vi "4ChNCS_BIOPAC_Zijing.vi"() -> ()   [LabVIEW 2016]
uses:
  <instrlib>/niUSRP/niUSRP Timestamp.ctl
  <vilib>/Utility/miscctls.llb/LVDateTimeRec.ctl
  <vilib>/Analysis/3filter.llb/Filter Passband Type.ctl
  <vilib>/sound2/lvsound2.llb/Sampling Mode.ctl
  <instrlib>/niUSRP/niUSRP Configure Time Start Trigger.vi
  <vilib>/Platform/browser.llb/Open URL in Default Browser (string).vi
  <instrlib>/niUSRP/niUSRP Write Tx Data (2D CDB).vi
  <instrlib>/niUSRP/niUSRP Fetch Rx Data (2D CDB).vi
  <vilib>/Analysis/3filter.llb/Butterworth Filter (DBL).vi
  <vilib>/Analysis/3filter.llb/Butterworth Filter (CDB).vi
  <vilib>/sound2/lvsound2.llb/Sound File Info (path).vi
  <vilib>/sound2/lvsound2.llb/Sound File Read Open.vi
  <vilib>/sound2/lvsound2.llb/Sound File Read (DBL).vi
  <vilib>/sound2/lvsound2.llb/Sound Output Write (DBL).vi
  <vilib>/measure/NI_MABase.lvlib
  <vilib>/Analysis/NI_AALBase.lvlib
  C:/Program Files (x86)/BIOPAC Systems, Inc/BIOPAC Hardware API 2.2 Education/x64/mpdev.dll
panel:
  in  "Mute":bool
  out "Play Sound":bool=TRUE
  in  "bottom filter":T1
  in  "top filter":T1=enum."Bandpass"
  out "Acq Started":bool
  out "# BIO View Q":i32
  out "# BIO Buffer":i32
  out "Boolean":bool=TRUE
  out "Disconnecting":bool
  out "Stopping":bool
  out "Connecting":bool
  out "Disconnected":bool
  in  "Show BIO":bool
  out "# BIOViewQ2":i32
  out "Array 1 View":dbl[](graph)
  out "Array 2 View":dbl[](graph)
  out "Array 3 View":dbl[](graph)
  out "Array 4 View":dbl[](graph)
  out "View Array Size":i32
  out "# Elements in Array":i32
  out "ACQ -# Elements":i32
  out "Receive Success":bool
  out "# ACQ cycles":i32
  out "Bytes Read":i32
  out "Bytes To Read":i32
  out "Receive Total Size":dbl format="%#_13g"
  out "Receiving":bool
  in  "Start Acquisition":bool
  in  "Disconnect":bool
  out "ACQ ms":dbl=250.0 format="%#_13g"
  in  "Stop Acquisition":bool
  out "Connected":bool
  in  "Sample Rate":dbl=1.0 caption="ms/sample" min=0.0
  in  "Analog Channels":i32[](array[numeric])=[1, 1, 1, 1]
  out "# Channels":dbl format="%#_13g"
  out "BIO Connect":i32
  in  "BIO Connect":bool=TRUE
  in  "OpenHTML":bool=TRUE
  in  "Abd (cm)":string="0"
  in  "Thorax (cm)":string="0"
  in  "Comments":string
  in  "Weight (lbs)":string="0"
  in  "Age (yrs)":string="0"
  in  "Sex":string(combo)="Female"
  in  "Height (cm)":string="0"
  in  "Case #":string="14"
  out "Start Time":T2
  out "Total Routine Time":dbl(slide) scale=0.0..300.0
  out "Elapsed Time":dbl caption="Elapsed Time (s)"
  out "Next Instruction":string
  out "Current Instruction":string
  in  "Routine Selection":T3(ring)
  out "Current Routine":string
  out "Tx3Rx4":dbl[](graph)
  out "Tx4Rx4":dbl[](graph)
  out "Tx4Rx3":dbl[](graph)
  out "Tx3Rx3":dbl[](graph)
  out "ChAmp":dbl[][](array[numeric])=[[1.7262327066457893e-05, 1.899698926539768e-05, 2.131979680782845e-05, 2.7507513862708948e-05, 3.236234947998919e-05, 3.384280863448985e-05, 3.3113712649913256e-05, 2.8744318806479064e-05, 2.4117959107532184e-05, 2.0714217164135817e-05, 1.7964639969242282e-05, 1.4127881869429752e-05, 1.5692535768228094e-05, 2.4152619914305532e-05, 2.8339686382715385e-05, 2.606906286720416e-05, 2.1755918570529384e-05, 2.0929028564145826e-05, 2.2419410493859248e-05, 2.1786896096171967e-05, 1.7145005999174206e-05, 1.5886785364638103e-05, 1.995380091360238e-05, 1.96084446445408e-05, 1.3881312052638574e-05, 5.368463432831762e-06, 7.886976522489036e-06, 1.718108126568357e-05, 1.984430714817916e-05, 1.8874058751572535e-05, 1.7869312672433515e-05, 1.7356735499504872e-05, 2.065235332503479e-05, 2.1951680154988656e-05, 2.0363547237431346e-05, 2.1229264430323524e-05, 2.188656276617781e-05, 2.1477411495382004e-05, 1.913194947952161e-05, 1.374906879007994e-05, 1.084407557924396e-05, 1.0538448835067238e-05, 1.3462486513328936e-05, 1.979383250422823e-05, 2.381539261154395e-05, 2.2167223174073578e-05, 1.7644503717147575e-05, 1.870536234643517e-05, 2.2751950524913166e-05, 2.340432192813861e-05, 2.2468849270761083e-05, 2.4188550691353842e-05, 2.7519058552290856e-05, 3.1102581077866726e-05, 3.580393911829494e-05, 3.78912649503874e-05, 3.327873597801261e-05, 2.4510981949940783e-05, 1.8465065354817837e-05, 1.7132224969133005e-05, 1.7642310138371268e-05, 1.88142956741822e-05, 1.560032046277488e-05, 9.753217862235494e-06, 1.2015090850038981e-05, 1.776834560720681e-05, 2.4803861691952522e-05, 2.8043624192078222e-05, 2.684382525540612e-05, 2.3530222840588965e-05, 2.0528849124310057e-05, 1.9668374613316667e-05, 1.9146637114645684e-05, 1.5474488036915515e-05, 1.739488550213199e-05, 2.5095299380068926e-05, 3.2858145215540916e-05, 3.439509649081835e-05, 2.6143868318774837e-05, 1.7977385637690134e-05, 1.6384181575586158e-05, 1.4888284293264162e-05, 1.1597491470576354e-05, 1.1445555578759772e-05, 1.4980688444081562e-05, 1.909173519498907e-05, 1.9461150455264684e-05, 1.845876729070065e-05, 1.8005010185132642e-05, 1.9028924898462435e-05, 1.7575955788217445e-05, 1.4184298105937452e-05, 9.414371560237339e-06, 5.4356042784590255e-06, 8.10928562517548e-06, 9.28876849225871e-06, 8.695785214389758e-06, 1.2695777397634576e-05, 1.6809431598631123e-05, 2.1908643727461497e-05], [0.39904903865563796, 0.39903176051530775, 0.39902405260596024, 0.3990221650023599, 0.3990182934858042, 0.39901299641778676, 0.39900459263010085, 0.39899398548309095, 0.3989851312683333, 0.3989817758172843, 0.39898441600096285, 0.3989920701551657, 0.3989957319087615, 0.3989970252526829, 0.3990014639144786, 0.3990082495650084, 0.39901677157837184, 0.39902202434845035, 0.3990170521098724, 0.3990061914814684, 0.39899957115083645, 0.39900163440594105, 0.39901134932465093, 0.3990245430143365, 0.3990299364956871, 0.3990206423396574, 0.39901294696264844, 0.399015237964853, 0.3990195320664335, 0.3990239908891069, 0.39902678858482366, 0.3990303142377581, 0.3990363654196349, 0.39903798034344395, 0.39903568308022536, 0.3990295778239386, 0.3990213145612541, 0.3990115641317417, 0.3990031911721688, 0.3990044335692754, 0.3990142055365442, 0.3990231880559529, 0.3990294810791408, 0.39903152543597487, 0.3990303417237137, 0.39902587131491124, 0.39902317862698444, 0.3990231908517323, 0.3990187535042287, 0.39901147460102687, 0.39900466569609977, 0.399000198693456, 0.398994572076958, 0.39898792975360287, 0.39898351183081265, 0.39898252129559103, 0.3989860199605185, 0.3989908704807006, 0.39899345184972185, 0.39899268675930705, 0.39898929894357515, 0.39898974479144206, 0.3989970434213525, 0.39900457970685, 0.3990084272376425, 0.3990059437407563, 0.39900092658003017, 0.3989998521554356, 0.3989999155043143, 0.39900335732390085, 0.3990086633280822, 0.39901161043288735, 0.3990153435576799, 0.3990232290578827, 0.39902895125044885, 0.3990233171970213, 0.39901091768095076, 0.3989963560226853, 0.3989823146041765, 0.39898013105698543, 0.39899131681473166, 0.3990088743561722, 0.39902163871137375, 0.39902552269435965, 0.3990216751013488, 0.3990108271690995, 0.3989999368161602, 0.39899179748001445, 0.3989869444795569, 0.3989823014007489, 0.3989811018380635, 0.3989866085692465, 0.3989974881575293, 0.399009653455826, 0.39902039237597164, 0.39903113834388676, 0.39903799466445666, 0.39903656085835637, 0.39902912933239515, 0.3990196685727854], [0.5089284260094796, 0.5089413529092005, 0.5089385924023097, 0.5089461735853302, 0.5089333321440155, 0.5089367652503622, 0.5089376331435306, 0.5089306671430541, 0.508949239645895, 0.5089486561361645, 0.5089529378833244, 0.5089419476875585, 0.5089298840108731, 0.5089475772042052, 0.5089441426339854, 0.5089427381450184, 0.5089483329108746, 0.5089280151098653, 0.5089336602793385, 0.5089062019851882, 0.5089074628030626, 0.5088932174425751, 0.5088701289561509, 0.5088760830698362, 0.5088683341509143, 0.5088818393635381, 0.5089000365985035, 0.5088962730652971, 0.5089053012825656, 0.5088919060061875, 0.5088858810710211, 0.5088778714303226, 0.508862396898039, 0.5088799706522465, 0.508890020250467, 0.5089068411749241, 0.508910151200762, 0.5088879724716624, 0.5088963605339264, 0.5088989546591678, 0.5089079531975655, 0.5089307483176185, 0.5089353690581762, 0.5089322510910641, 0.5089226818391756, 0.5089231205950179, 0.5089421889187917, 0.5089302121637822, 0.5089288553338916, 0.5089136387417116, 0.5088923938634197, 0.5088806790242092, 0.5088543127997475, 0.5088388632427274, 0.5088290815518671, 0.5088136498514574, 0.508828716232115, 0.5088373004254244, 0.5088536031198835, 0.5088663652543981, 0.5088663647379902, 0.5088663839922184, 0.5088589552438861, 0.5088642449634635, 0.5088725023266256, 0.5088718014416865, 0.5088674063260687, 0.5088515437004615, 0.5088682831786894, 0.5088713788197812, 0.5088809924897628, 0.508878513506942, 0.5088771181893693, 0.5088848435184512, 0.5088770842370816, 0.5088914766511436, 0.5089003523667647, 0.5089066301516674, 0.5089314320882471, 0.5089402101447223, 0.508962553406896, 0.5089753861787446, 0.5089593307295952, 0.5089478542324088, 0.5089278310589712, 0.5089248500720587, 0.5089163513653545, 0.5089005689237424, 0.5089083211616405, 0.5088993300683022, 0.5088927412237987, 0.5088830866377116, 0.5088718481995638, 0.5088897909905771, 0.5088809733102648, 0.5088790935282286, 0.5088680814653207, 0.5088523600270333, 0.5088613943195607, 0.5088543176402154], [2.0662941946213977e-05, 2.282608405319783e-05, 2.237600508813514e-05, 2.2542693256186783e-05, 2.041826329305299e-05, 1.6288400811782785e-05, 1.0891495139698275e-05, 1.4190599881567273e-05, 1.8742691366266016e-05, 1.8736119036749436e-05, 1.741774537028846e-05, 1.5658954058158222e-05, 1.5904856683822096e-05, 1.6871005066910787e-05, 1.5599249074465836e-05, 1.3520520470394872e-05, 1.3927163947888679e-05, 1.5334805249818678e-05, 1.4564830067379515e-05, 9.817520346860189e-06, 1.3098820613974226e-05, 1.929550220456421e-05, 2.3072255815616586e-05, 2.4321951176986116e-05, 2.3250917563816834e-05, 2.1644284217119052e-05, 1.7041306350033735e-05, 1.0688883027066213e-05, 9.28433634468159e-06, 1.1420718289762068e-05, 1.7056250213804775e-05, 1.9836991189555113e-05, 1.746716828521344e-05, 1.2441527630540996e-05, 8.566795426917848e-06, 9.815076354382859e-06, 1.0229272880058857e-05, 9.936691802926115e-06, 1.536494187514889e-05, 2.3346259934086635e-05, 2.7477587888222747e-05, 2.882421007601368e-05, 2.763067836551142e-05, 2.1577345489474273e-05, 1.3485424327083916e-05, 9.52579824483287e-06, 1.3113651673496717e-05, 1.5276095683726537e-05, 1.6308973250379756e-05, 1.8045078515596545e-05, 1.7849042225306495e-05, 1.2607829522468473e-05, 7.109107971268437e-06, 6.6038815895810515e-06, 6.924972052119899e-06, 4.965235247536195e-06, 5.757305113334596e-06, 9.21497446069365e-06, 9.781248515919794e-06, 1.0683021318304504e-05, 1.196938592791573e-05, 1.159802409297526e-05, 1.012272777630437e-05, 9.65935822948268e-06, 1.4116839432017005e-05, 1.847684147148342e-05, 1.6783927528588872e-05, 1.0863513026975652e-05, 7.650914818223192e-06, 9.456183557358687e-06, 1.0426180609097815e-05, 8.567604650724215e-06, 8.546559610017728e-06, 1.2946532793024891e-05, 1.7245567743458815e-05, 2.0097444147186203e-05, 2.0459407417437442e-05, 1.9957232554286306e-05, 1.996659645997603e-05, 1.7332136966233293e-05, 1.5115608112097958e-05, 1.762095864401886e-05, 1.992020410454883e-05, 2.0585166404108466e-05, 2.212056735942569e-05, 2.2957279986002272e-05, 2.3103396847026532e-05, 2.320807116373638e-05, 2.0818984342366494e-05, 1.789850158592137e-05, 1.64936985167028e-05, 1.4204813599995013e-05, 1.2878752736428332e-05, 1.4757379916553103e-05, 1.713867099725903e-05, 1.6105166890214558e-05, 1.20593443919334e-05, 1.2171370167939264e-05, 1.2336933066341984e-05, 1.1620987924410626e-05]]
  out "Output":bool=TRUE
  out "Ch4 Amplitude":dbl step=0.05 format="%#.6g"
  out "Ch3 Amplitude":dbl=0.25 step=0.05 format="%#.6g"
  out "Ch2 Amplitude":dbl=0.6 step=0.05 format="%#.6g"
  out "Ch1 Amplitude":dbl step=0.05 format="%#.6g"
  out "Tx1Rx2":dbl[](graph)
  out "Tx2Rx2":dbl[](graph)
  out "Tx2Rx1":dbl[](graph)
  out "Dis Sampling Rate":dbl=1000.0 format="%#_6p"
  in  "DownSamplingRatio 2":i32=10
  out "Sampling Rate":dbl=10000.0 format="%#_6p"
  out "Flush":bool
  out "8 Ch Heart":dbl[][](array[numeric])
  out "NCS Save Loops":i32=56132
  out "Save":bool
  out "# NCS Buffer":i32
  out "Buffer":bool
  in  "fl Bottom":dbl=10.0 format="%0.4f"
  in  "fh Bottom":dbl=20.0 format="%0.2f"
  in  "DownSamplingRatio1":i32=100
  in  "fl Top":dbl=4.0 format="%0.4f"
  in  "fh Top":dbl=20.0 format="%0.2f"
  out "# elements in view queue":i32
  out "Tx1Rx1":dbl[](graph)
  out "DownSamplingRatio":i32=100
  out "BW/2":dbl=1000.0
  out "# IQ queue Ch 2":i32
  out "# IQ queue Ch 1":i32
  in  "Dis2":bool=TRUE
  in  "Dis1":bool=TRUE
  out "IQ Graph 2":dbl[][](graph)
  out "IQ Graph":dbl[][](graph)
  out "Tx2 Waveform":cdb[][](array[numeric])
  out "Tx1 Waveform":cdb[][](array[numeric])
  in  "Ch3&4 carrier frequency [Hz] 2":dbl=1000000000.0 format="%#_6p"
  in  "Ch1&2 carrier frequency [Hz]":dbl=900000000.0 format="%#_6p"
  in  "Rx2 Gain 2":dbl=15.0 format="%#_6f"
  in  "Tx2 Gain 2":dbl=20.0 format="%#_6f"
  in  "Rx1 Gain 2":dbl=15.0 format="%#_6f"
  in  "Tx1 Gain 2":dbl=20.0 format="%#_6f"
  out "error out 2":errorcluster
  in  "Start Trigger Time 2":T4={"whole seconds"=1, "fractional seconds"=0.0}
  in  "Channel 4 Tone Amplitude":dbl=0.5 step=0.05 format="%#.6g"
  in  "Channel 4 Tone Frequency":dbl=430000.0 format="%#_6p"
  in  "Channel 3 Tone Amplitude":dbl=0.5 step=0.05 format="%#.6g"
  in  "Channel 3 Tone Frequency":dbl=473000.0 format="%#_6p"
  out "Tx2 Waveform Graph":waveform(dbl)[](graph)=[{"t0"=timestamp(0.45999999999999996 s since 1904-01-01), "dt"=1e-06, "Y"=array[10000 elements]}, {"t0"=timestamp(0.45999999999999996 s since 1904-01-01), "dt"=1e-06, "Y"=array[10000 elements]}, {"t0"=timestamp(0.45999999999999996 s since 1904-01-01), "dt"=1e-06, "Y"=array[10000 elements]}, {"t0"=timestamp(0.45999999999999996 s since 1904-01-01), "dt"=1e-06, "Y"=array[10000 elements]}]
  in  "Waveform Size 2":dbl=10000.0
  in  "Stop 2":bool
  in  "Device Name 2":refnum<k15>="MyB210_2"
  in  "Tx2 Gain 1":dbl=20.0 format="%#_6f"
  in  "Tx IQ Rate 2":dbl=1000000.0 format="%#_6p"
  in  "Rx2 Gain 1":dbl=15.0 format="%#_6f"
  in  "Rx IQ Rate 2":dbl=1000000.0 format="%#_6p"
  out "error out 1":errorcluster
  in  "Start Trigger Time":T4={"whole seconds"=1, "fractional seconds"=0.0}
  in  "Stop":bool
  in  "Channel 2 Tone Amplitude":dbl=0.5 step=0.05 format="%#.6g"
  in  "Channel 2 Tone Frequency":dbl=440000.0 format="%#_6p"
  in  "Channel 1 Tone Amplitude":dbl=0.5 step=0.05 format="%#.6g"
  in  "Channel 1 Tone Frequency":dbl=355000.0 format="%#_6p"
  out "Tx1 Waveform Graph":waveform(dbl)[](graph)=[{"t0"=timestamp(0.45999999999999996 s since 1904-01-01), "dt"=1e-06, "Y"=array[10000 elements]}, {"t0"=timestamp(0.45999999999999996 s since 1904-01-01), "dt"=1e-06, "Y"=array[10000 elements]}, {"t0"=timestamp(0.45999999999999996 s since 1904-01-01), "dt"=1e-06, "Y"=array[10000 elements]}, {"t0"=timestamp(0.45999999999999996 s since 1904-01-01), "dt"=1e-06, "Y"=array[10000 elements]}]
  in  "Waveform Size 1":dbl=10000.0
  in  "Device Name":refnum<k15>="MyB210_1"
  in  "Tx1 Gain 1":dbl=20.0 format="%#_6f"
  in  "Tx IQ Rate 1":dbl=1000000.0 format="%#_6p"
  in  "Rx1 Gain 1":dbl=15.0 format="%#_6f"
  in  "Rx IQ Rate 1":dbl=1000000.0 format="%#_6p"
  # "Misc"
  # "Tx Waveform"
  # "IQ waveform"
  # "NCS"
  # "Channel Settings"
  # "Channel 1"
  # "Device Settings"
  # "BIO"
  # "Channel 2"
  # "Filters"
  # "Buffers"
  # "BIOPAC Connection"
  # "Channel 3"
  # "Post Study Survey:"
  # "https://cornell.qualtrics.com/jfe/form/SV_9QryoqkUKquSXD7"
  # "Channel 4"
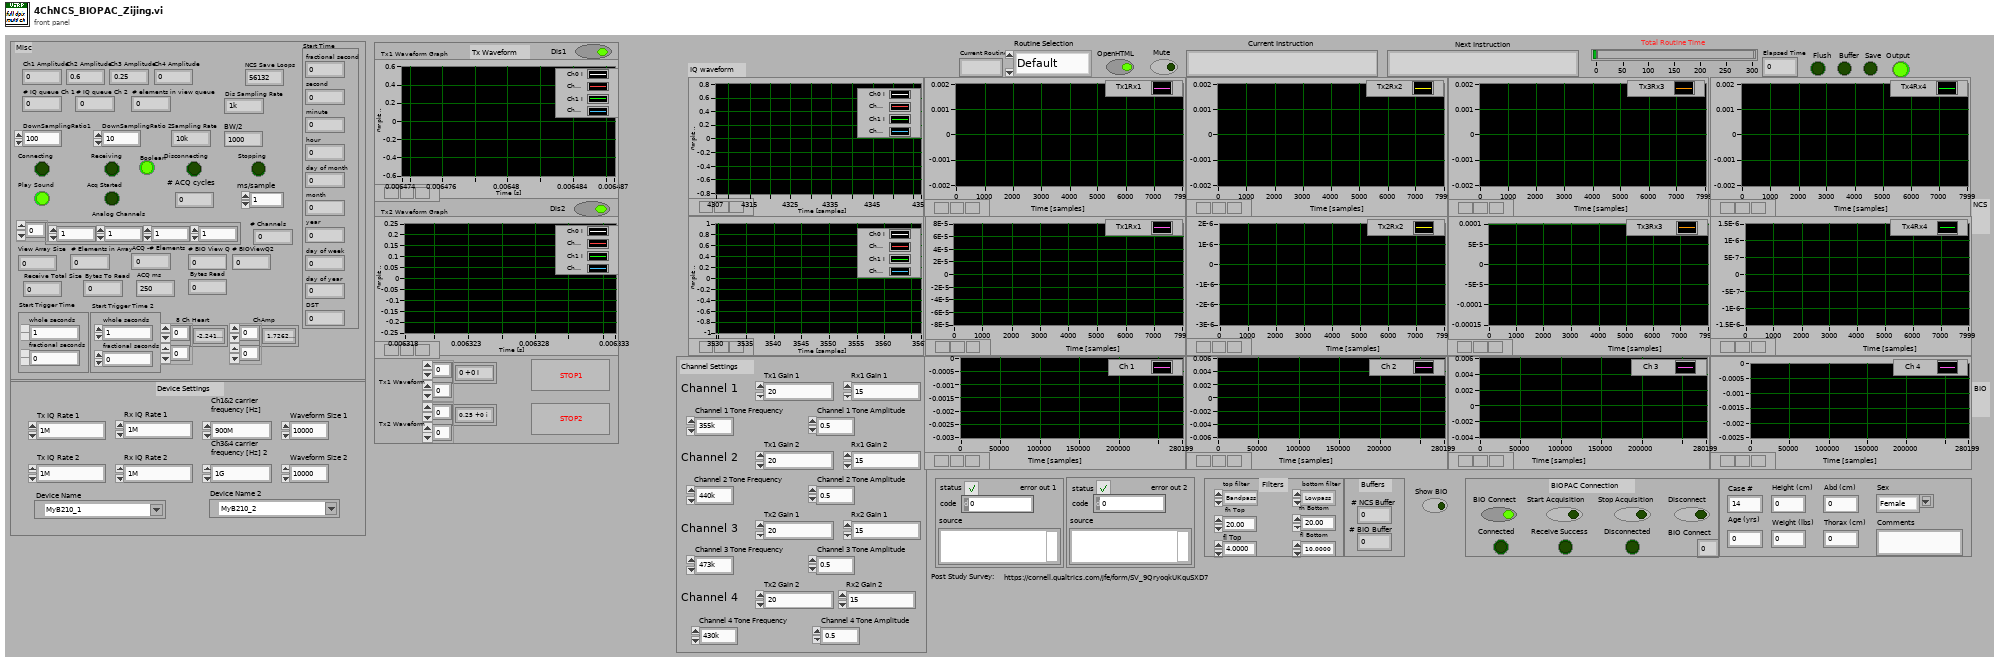
[diagram p1: front panel]
types:
  T1 = typedef "NI_AALBase.lvlib/Filter Passband Type.ctl" = enum32{"Lowpass", "Highpass", "Bandpass", "Bandstop"}
  T2 = typedef "LVDateTimeRec.ctl" = cluster{"fractional second":dbl, "second":i32, "minute":i32, "hour":i32, "day of month":i32, "month":i32, "year":i32, "day of week":i32, "day of year":i32, "DST":i32}
  T3 = enum16{"Default", "Test Run", "Training", "Routine 1", "Routine 2", "Routine 3", "Routine 4", "Routine 5a", "Routine 5b"}
  T4 = typedef "niUSRP Timestamp.ctl" = cluster{"whole seconds":u64, "fractional seconds":dbl}
  T5 = typedef "Sampling Mode.ctl" = i32
  T6 = typedef "Sound Data Format.ctl" = cluster{"sample rate (S/s)":dbl, "number of channels":i32, "bits per sample":i32}
  T7 = typedef "Sound File Refnum.ctl" = refnum<file>
  T8 = typedef "Sound Output Task ID.ctl" = u32
  T9 = enum16{"open", "open or create", "create or replace", "create", "open (read-only)"}
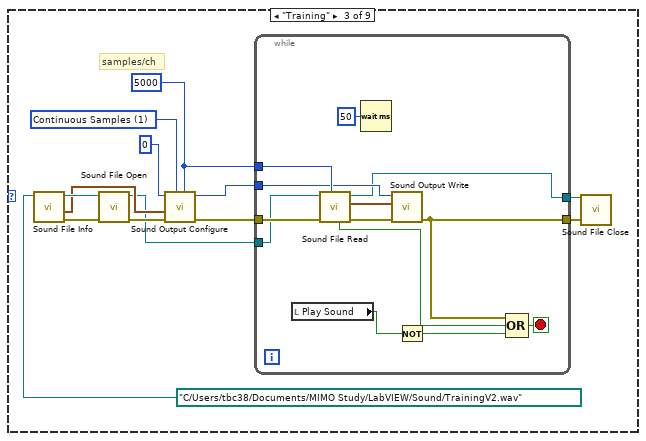
[diagram p4: hidden frame]
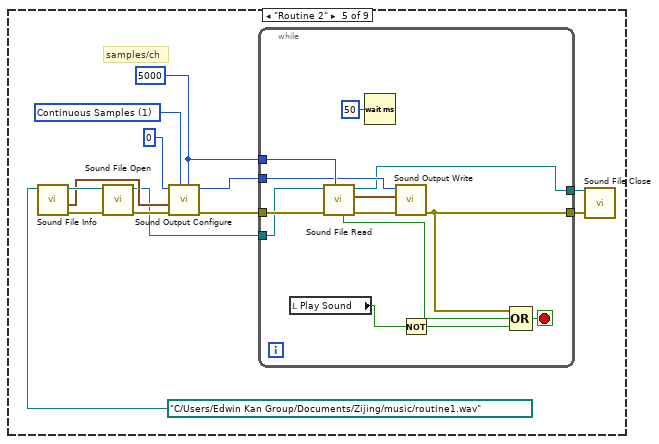
[diagram p6: hidden frame]
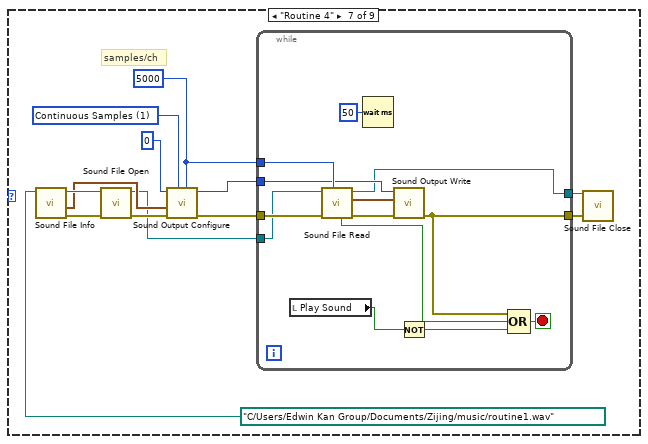
[diagram p8: hidden frame]
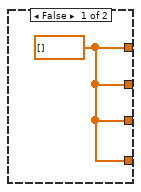
[diagram p11: hidden frame]
diagram:
  w1 = FALSE
  w29 = enum16{"Default"}."Default"
  w26 = 0.0 ("element")
  w27 = 800 ("dimension size")
  w33 = 4 ("dimension size")
  (unwired) 10
  w85 = "RX2"  # Tx active antenna
  w86 = "RX2"  # Tx active antenna
  w142 = 1 items=["Now", "Next Timebase Edge"] ("apply timestamp")
  w114 = "TX1"  # Tx active antenna
  w208 = 1 items=["Now", "Next Timebase Edge"] ("apply timestamp")
  w180 = "TX1"  # Tx active antenna
  # "Sound"
  # "Get it so that it acquires the proper number of cycles for the routine time. Front should be save synchronized"
  # "BIOPAC QUEUE"
  # "Current Sync Method:\nStart Buffering as soon as Acquisition Starts"
  # "Biopac Code. Use the flags to switch between these loops.\nCONNECT- Run to connect to the BIOPAC. Acquisition will not start. 'Connect Success' returns the status of this function.\nSTART ACQUISITION- Run to begin acquiring data from the BIOPAC. SYNCHRONIZATION IS IMPORTANT HERE.\nSTOP ACQUISITION- Run to stop acquiring data. The BIOPAC will disconnect and reconnect to prepare for another acquisition.\nDISCONNECT- Run to disconnect from BIOPAC. This will prohibit connection until the VI is restarted.\nSHOW/VIEWING- Dequeues the elements and displays them."
  # "Routine selection and implementation Loop"
  # "DownSamplingRatio"
  # "Set the attributes \nspecific to channel 1."
  # "Set the attributes \nspecific to channel 0."
  # "Set the attributes \nused by both Rx channels"
  # "Set the attributes \nspecific to Rx channel 1."
  # "Set the attributes \nspecific to Rx channel 0."
  # "Set the attributes \nspecific to channel 1."
  # "Set the attributes \nspecific to channel 0."
  # "Set the attributes \nused by both Rx channels"
  # "Set the attributes \nspecific to Rx channel 1."
  # "Set the attributes \nspecific to Rx channel 0."
  n1 = local write "BIO Connect"(w1) -> ()
  n2 = local write "Start Acquisition"(w1) -> ()
  n3 = local write "Stop Acquisition"(w1) -> ()
  n4 = local write "Disconnect"(w1) -> ()
  n5 = local write "Show BIO"(w1) -> ()
  n6 = local read "Device Name 2"() -> (w150:refnum<k15>)
  n7 = while {
    stop <- FALSE stop-if-true
    n8 = Wait (ms)(milliseconds to wait=50) -> ()  [unwired: 1 out]
    n9 = Not(x="Mute") -> (.not. x?=w224:bool)
    n10 = case shown="True" w224 {
      frame False {
      }
      frame True {
        n11 = local read "Routine Selection"() -> (w227:T3)
        n12 = case shown="\"Default\", Default" w227 {
          frame "Default", Default {
          }
          frame "Test Run" {
          }
          frame "Training" {
            w231 = 5000
            w234 = T5 1 items=["Finite Samples", "Continuous Samples"] ("sample mode")
            # "samples/ch"
            n13 = call-poly <vilib>:"Sound File Info.vi"("path"=path "C:/Users/tbc38/Documents/MIMO Study/LabVIEW/Sound/TrainingV2.wav") -> ("error out"=w239:errorcluster, "sound format"=w235:T6, "path out"=w240:path)  [unwired: 7 in, 1 out]
            n14 = call-poly <vilib>:"Sound File Open.vi"("error in (no error)"=w239, "path"=w240) -> ("error out"=w238:errorcluster, "sound file refnum"=w230:T7)  [unwired: 8 in]
            n15 = call <vilib>:"Sound Output Configure.vi"("number of samples/ch"=w231, "sample mode"=w234, "error in (no error)"=w238, "sound format"=w235, "device ID"=u32 0) -> ("error out"=w233:errorcluster, "task ID"=w232:T8)  [unwired: 5 in]
            n16 = while {
              tunnel: w233 -> [w251]
              tunnel: w232 -> [w252]
              tunnel: w231 -> [w253]
              tunnel: w230 -> [w250]
              tunnel: [w244] -> w229
              tunnel: [w248] -> w228
              stop <- w242 stop-if-true
              n17 = local read "Play Sound"() -> (w241:bool)
              n18 = call-poly <vilib>:"Sound File Read.vi"("number of samples/ch (-1: all)"=w253, "error in (no error)"=w251, "sound file refnum"=w250) -> ("error out"=w247:errorcluster, "data"=w246:waveform(dbl)[], "sound file refnum out"=w248:T7, "end of file?"=w245:bool)  [unwired: 4 in, 1 out]
              n19 = Wait (ms)(milliseconds to wait=50) -> ()  [unwired: 1 out]
              n20 = call-poly <vilib>:"Sound Output Write.vi"("error in (no error)"=w247, "data"=w246, "task ID"=w252) -> ("error out"=w244:errorcluster)  [unwired: 7 in, 1 out]
              n21 = Not(x=w241) -> (.not. x?=w243:bool)
              n22 = Compound Arithmetic op=OR(w244, w245, w243) -> (w242:bool)
            }
            n23 = call <vilib>:"Sound File Close.vi"("error in (no error)"=w229, "sound file refnum"=w228) -> ()  [unwired: 9 in, 1 out]
          }
          frame "Routine 1" {
          }
          frame "Routine 2" {
            w257 = 5000
            w260 = T5 1 items=["Finite Samples", "Continuous Samples"] ("sample mode")
            # "samples/ch"
            n24 = call-poly <vilib>:"Sound File Info.vi"("path"=path "C:/Users/Edwin Kan Group/Documents/Zijing/music/routine1.wav") -> ("error out"=w265:errorcluster, "sound format"=w261:T6, "path out"=w266:path)  [unwired: 7 in, 1 out]
            n25 = call-poly <vilib>:"Sound File Open.vi"("error in (no error)"=w265, "path"=w266) -> ("error out"=w264:errorcluster, "sound file refnum"=w256:T7)  [unwired: 8 in]
            n26 = call <vilib>:"Sound Output Configure.vi"("number of samples/ch"=w257, "sample mode"=w260, "error in (no error)"=w264, "sound format"=w261, "device ID"=u32 0) -> ("error out"=w259:errorcluster, "task ID"=w258:T8)  [unwired: 5 in]
            n27 = while {
              tunnel: w259 -> [w277]
              tunnel: w258 -> [w278]
              tunnel: w257 -> [w279]
              tunnel: w256 -> [w276]
              tunnel: [w270] -> w255
              tunnel: [w274] -> w254
              stop <- w268 stop-if-true
              n28 = local read "Play Sound"() -> (w267:bool)
              n29 = call-poly <vilib>:"Sound File Read.vi"("number of samples/ch (-1: all)"=w279, "error in (no error)"=w277, "sound file refnum"=w276) -> ("error out"=w273:errorcluster, "data"=w272:waveform(dbl)[], "sound file refnum out"=w274:T7, "end of file?"=w271:bool)  [unwired: 4 in, 1 out]
              n30 = Wait (ms)(milliseconds to wait=50) -> ()  [unwired: 1 out]
              n31 = call-poly <vilib>:"Sound Output Write.vi"("error in (no error)"=w273, "data"=w272, "task ID"=w278) -> ("error out"=w270:errorcluster)  [unwired: 7 in, 1 out]
              n32 = Not(x=w267) -> (.not. x?=w269:bool)
              n33 = Compound Arithmetic op=OR(w270, w271, w269) -> (w268:bool)
            }
            n34 = call <vilib>:"Sound File Close.vi"("error in (no error)"=w255, "sound file refnum"=w254) -> ()  [unwired: 9 in, 1 out]
          }
          frame "Routine 3" {
          }
          frame "Routine 4" {
            w283 = 5000
            w286 = T5 1 items=["Finite Samples", "Continuous Samples"] ("sample mode")
            # "samples/ch"
            n35 = call-poly <vilib>:"Sound File Info.vi"("path"=path "C:/Users/Edwin Kan Group/Documents/Zijing/music/routine1.wav") -> ("error out"=w291:errorcluster, "sound format"=w287:T6, "path out"=w292:path)  [unwired: 7 in, 1 out]
            n36 = call-poly <vilib>:"Sound File Open.vi"("error in (no error)"=w291, "path"=w292) -> ("error out"=w290:errorcluster, "sound file refnum"=w282:T7)  [unwired: 8 in]
            n37 = call <vilib>:"Sound Output Configure.vi"("number of samples/ch"=w283, "sample mode"=w286, "error in (no error)"=w290, "sound format"=w287, "device ID"=u32 0) -> ("error out"=w285:errorcluster, "task ID"=w284:T8)  [unwired: 5 in]
            n38 = while {
              tunnel: w285 -> [w303]
              tunnel: w284 -> [w304]
              tunnel: w283 -> [w305]
              tunnel: w282 -> [w302]
              tunnel: [w296] -> w281
              tunnel: [w300] -> w280
              stop <- w294 stop-if-true
              n39 = local read "Play Sound"() -> (w293:bool)
              n40 = call-poly <vilib>:"Sound File Read.vi"("number of samples/ch (-1: all)"=w305, "error in (no error)"=w303, "sound file refnum"=w302) -> ("error out"=w299:errorcluster, "data"=w298:waveform(dbl)[], "sound file refnum out"=w300:T7, "end of file?"=w297:bool)  [unwired: 4 in, 1 out]
              n41 = Wait (ms)(milliseconds to wait=50) -> ()  [unwired: 1 out]
              n42 = call-poly <vilib>:"Sound Output Write.vi"("error in (no error)"=w299, "data"=w298, "task ID"=w304) -> ("error out"=w296:errorcluster)  [unwired: 7 in, 1 out]
              n43 = Not(x=w293) -> (.not. x?=w295:bool)
              n44 = Compound Arithmetic op=OR(w296, w297, w295) -> (w294:bool)
            }
            n45 = call <vilib>:"Sound File Close.vi"("error in (no error)"=w281, "sound file refnum"=w280) -> ()  [unwired: 9 in, 1 out]
          }
          frame "Routine 5a" {
          }
          frame "Routine 5b" {
          }
        }
      }
    }
  }
  n46 = while {
    stop <- FALSE stop-if-true
    # "STOP ACQUISITION"
    n47 = local read "Connected"() -> (w310:bool)
    n48 = local read "Receiving"() -> (w309:bool)
    n49 = local read "Stopping"() -> (w307:bool)
    n50 = Wait (ms)(milliseconds to wait=100) -> ()  [unwired: 1 out]
    n51 = Not(x=w307) -> (.not. x?=w306:bool)
    n52 = And(x=w309, y=w306) -> (x .and. y?=w308:bool)
    n53 = And(x=w310, y=w308) -> (x .and. y?=w311:bool)
    n54 = And(x="Stop Acquisition", y=w311) -> (x .and. y?=w314:bool)
    n55 = case shown="True" w314 {
      frame False {
      }
      frame True {
        n56 = flat-sequence {
          frame #0 {
            n57 = local write "Stopping"(TRUE) -> ()
            n58 = dll-call lib="C:/Program Files (x86)/BIOPAC Systems, Inc/BIOPAC Hardware API 2.2 Education/x64/mpdev.dll" fn="stopAcquisition" label="stop"() -> ()  [unwired: 4 in, 2 out]
            n59 = local write "Receiving"(FALSE) -> ()
          }
          frame #1 {
            n60 = dll-call lib="C:/Program Files (x86)/BIOPAC Systems, Inc/BIOPAC Hardware API 2.2 Education/x64/mpdev.dll" fn="disconnectMPDev" label="disconnect"() -> ()  [unwired: 4 in, 2 out]
          }
          frame #2 {
            n61 = local read "ACQ ms"() -> (w319:dbl)
            n62 = Add(x=w319, y=200) -> (x+y=w320:dbl)
            n63 = Wait (ms)(milliseconds to wait=w320) -> ()  [unwired: 1 out]
          }
          frame #3 {
            w321 = FALSE
            n64 = local write "Stop Acquisition"(w321) -> ()
            n65 = local write "Stopping"(w321) -> ()
            n66 = local write "Connected"(w321) -> ()
            n67 = local write "Receive Success"(w321) -> ()
          }
        }
      }
    }
  }
  n68 = while {
    stop <- FALSE stop-if-true
    # "CONNECT"
    n69 = local read "Connecting"() -> (w330:bool)
    n70 = local read "Connected"() -> (w329:bool)
    n71 = local read "Disconnected"() -> (w326:bool)
    n72 = Wait (ms)(milliseconds to wait=500) -> ()  [unwired: 1 out]
    n73 = Not(x=w330) -> (.not. x?=w328:bool)
    n74 = Not(x=w329) -> (.not. x?=w325:bool)
    n75 = Not(x=w326) -> (.not. x?=w324:bool)
    n76 = And(x=w325, y=w324) -> (x .and. y?=w323:bool)
    n77 = And(x=w328, y=w323) -> (x .and. y?=w327:bool)
    n78 = And(x="BIO Connect", y=w327) -> (x .and. y?=w331:bool)
    n79 = case shown="True" w331 {
      frame False {
      }
      frame True {
        n80 = flat-sequence {
          frame #0 {
            n81 = local write "BIO Connect"(FALSE) -> ()
            n82 = local write "Connecting"(TRUE) -> ()
          }
          frame #1 {
            w341 = u32 1  # MPSUCCESS
            w350 = 10  # Enumeration Value For USB
            w349 = 103  # Enumeration Value for MP36
            n83 = String To Byte Array(string="") -> (unsigned byte array=w347:u8[])
            n84 = dll-call lib="C:/Program Files (x86)/BIOPAC Systems, Inc/BIOPAC Hardware API 2.2 Education/x64/mpdev.dll" fn="connectMPDev" label="connect"("mptype"=w349, "mpcomtype"=w350, "sn"=w347) -> ("return type"=w346:u32)  [unwired: 6 in, 2 out]
            "BIO Connect" <- w346
            n85 = Not Equal?(x=w346, y=w341) -> (x != y?=w345:bool)
            n86 = case shown="True" w345 {
              frame False {
              }
              frame True {
                n87 = flat-sequence {
                  frame #0 {
                    n88 = dll-call lib="C:/Program Files (x86)/BIOPAC Systems, Inc/BIOPAC Hardware API 2.2 Education/x64/mpdev.dll" fn="stopAcquisition" label="stop"() -> ()  [unwired: 4 in, 2 out]
                  }
                  frame #1 {
                    n89 = dll-call lib="C:/Program Files (x86)/BIOPAC Systems, Inc/BIOPAC Hardware API 2.2 Education/x64/mpdev.dll" fn="disconnectMPDev" label="disconnect"() -> ()  [unwired: 4 in, 2 out]
                  }
                }
              }
            }
            n90 = Not(x=w345) -> (.not. x?=w344:bool)
            n91 = case shown="True" w344 {
              tunnel: [w351 w353] -> w342
              tunnel: [w351 w352] -> w343
              frame False {
                w351 = 0
              }
              frame True {
                n92 = flat-sequence {
                  tunnel: [w357] -> w353
                  tunnel: [w359] -> w352
                  frame #0 {
                    n93 = To Double Precision Float(number="Analog Channels") -> (double precision float=w355:dbl[])
                    n94 = Add Array Elements(numeric array=w355) -> (sum=→"# Channels":dbl)
                    n95 = dll-call lib="C:/Program Files (x86)/BIOPAC Systems, Inc/BIOPAC Hardware API 2.2 Education/x64/mpdev.dll" fn="setAcqChannels" label="set analog CH"("aCH"="Analog Channels") -> ("return type"=w357:u32)  [unwired: 4 in, 2 out]
                  }
                  frame #1 {
                    n96 = dll-call lib="C:/Program Files (x86)/BIOPAC Systems, Inc/BIOPAC Hardware API 2.2 Education/x64/mpdev.dll" fn="setSampleRate" label="set sample rate"("rate"="Sample Rate") -> ("return type"=w359:u32)  [unwired: 4 in, 2 out]
                  }
                }
              }
            }
            n97 = Not Equal?(x=w343, y=w341) -> (x != y?=w338:bool)
            n98 = Not Equal?(x=w342, y=w341) -> (x != y?=w337:bool)
            n99 = Not(x=w337) -> (.not. x?=w339:bool)
            n100 = case shown="True" w337 {
              frame False {
              }
              frame True {
                n101 = flat-sequence {
                  frame #0 {
                    n102 = dll-call lib="C:/Program Files (x86)/BIOPAC Systems, Inc/BIOPAC Hardware API 2.2 Education/x64/mpdev.dll" fn="stopAcquisition" label="stop"() -> ()  [unwired: 4 in, 2 out]
                  }
                  frame #1 {
                    n103 = dll-call lib="C:/Program Files (x86)/BIOPAC Systems, Inc/BIOPAC Hardware API 2.2 Education/x64/mpdev.dll" fn="disconnectMPDev" label="disconnect"() -> ()  [unwired: 4 in, 2 out]
                  }
                }
              }
            }
            n104 = case shown="True" w338 {
              frame False {
              }
              frame True {
                n105 = flat-sequence {
                  frame #0 {
                    n106 = dll-call lib="C:/Program Files (x86)/BIOPAC Systems, Inc/BIOPAC Hardware API 2.2 Education/x64/mpdev.dll" fn="stopAcquisition" label="stop"() -> ()  [unwired: 4 in, 2 out]
                  }
                  frame #1 {
                    n107 = dll-call lib="C:/Program Files (x86)/BIOPAC Systems, Inc/BIOPAC Hardware API 2.2 Education/x64/mpdev.dll" fn="disconnectMPDev" label="disconnect"() -> ()  [unwired: 4 in, 2 out]
                  }
                }
              }
            }
            n108 = Not(x=w338) -> (.not. x?=w340:bool)
            n109 = And(x=w340, y=w339) -> (x .and. y?=w336:bool)
            n110 = local write "Connected"(w336) -> ()
          }
          frame #2 {
            n111 = local write "Connecting"(FALSE) -> ()
          }
        }
      }
    }
  }
  n112 = local read "Device Name"() -> (w216:refnum<k15>)
  n113 = call <instrlib>:"niUSRP Open Rx Session.vi"("device names"="Device Name 2") -> ("session handle out"=w141:refnum<k15>, "error out"=w140:errorcluster)  [unwired: 13 in]
  n114 = property class="niUSRP"(reference=w141, error in=w140, "Enabled Channels"="0,1" ("Configuration:Enabled Channels")) -> (reference out=w139:refnum<k15>, error out=w138:errorcluster)
  n115 = call <instrlib>:"niUSRP Open Rx Session.vi"("device names"="Device Name") -> ("session handle out"=w207:refnum<k15>, "error out"=w206:errorcluster)  [unwired: 13 in]
  n116 = property class="niUSRP"(reference=w207, error in=w206, "Enabled Channels"="0,1" ("Configuration:Enabled Channels")) -> (reference out=w205:refnum<k15>, error out=w204:errorcluster)
  n117 = call-poly <instrlib>:"niUSRP Configure Trigger.vi"("session handle"=w139, "start trigger time"="Start Trigger Time 2", "error in (no error)"=w138) -> ("session handle out"=w135:refnum<k15>, "error out"=w134:errorcluster)  [unwired: 11 in]
  n118 = call-poly <instrlib>:"niUSRP Configure Trigger.vi"("session handle"=w205, "start trigger time"="Start Trigger Time", "error in (no error)"=w204) -> ("session handle out"=w201:refnum<k15>, "error out"=w200:errorcluster)  [unwired: 11 in]
  n119 = property class="niUSRP"(reference=w135, error in=w134, "IQ Rate"="Rx IQ Rate 2") -> (reference out=w131:refnum<k15>, error out=w132:errorcluster)
  n120 = property class="niUSRP"(reference=w201, error in=w200, "IQ Rate"="Rx IQ Rate 1") -> (reference out=w197:refnum<k15>, error out=w198:errorcluster)
  n121 = property class="niUSRP" props=["Model", "Reference Frequency Source", "Timebase Clock Source"](reference=w197, error in=w198, "Reference Frequency Source"="RefIn" ("Clocking and Synchronization:Reference Frequency Source"), "Timebase Clock Source"="PpsIn" ("Clocking and Synchronization:Timebase Clock Source")) -> (reference out=w193:refnum<k15>, error out=w194:errorcluster)  [unwired: 1 out]
  n122 = property class="niUSRP" props=["Model", "Reference Frequency Source", "Timebase Clock Source"](reference=w131, error in=w132, "Reference Frequency Source"="RefIn" ("Clocking and Synchronization:Reference Frequency Source"), "Timebase Clock Source"="PpsIn" ("Clocking and Synchronization:Timebase Clock Source")) -> (reference out=w127:refnum<k15>, error out=w128:errorcluster)  [unwired: 1 out]
  n123 = local write "Routine Selection"(w29) -> ()
  n124 = local read "# Channels"() -> (w4:dbl)
  n125 = local read "ACQ ms"() -> (w3:dbl)
  n126 = while {
    shift-right: ["Routine Selection"] -> _
    shift-left: w29 -> [w367]
    stop <- FALSE stop-if-true
    n127 = case shown="\"Routine 5a\"" w367 {
      tunnel: ["Default" w397 "Isovolumetric Training" "Routine1" "Routine2" "Routine3" "Routine4" "Routine5a" "Routine5b"] -> w368
      tunnel: [w383 w397 w406 "normal breathing+speaking" "normal breathing+eating" " exercise" "exercise " "normal breathing+straw" "end"] -> w365
      tunnel: [w370 _ w404 w452 w474 w507 w525 w551 w569] -> w363
      tunnel: [w370 _ w404 w452 w474 w507 w525 w551 w569] -> w364
      tunnel: [w383 w397 w405 " normal breathing" "normal breathing+ speaking" "post-exercise normal breathing" "post exercise -breathing protocol" "normal breathing+mask" "normal breathing with straw"] -> w362
      tunnel: [w382 w396 w403 w450 w479 w505 w530 w554 w573] -> w361
      frame "Default" {
        w370 = 0.0
        w383 = "No instruction"
        # "BIO should not be acquiring"
        # "If BIO is not connected, attempt to reconnect"
        n128 = Seconds To Date/Time(time stamp (now)=0.0) -> (date time rec=w382:T2)  [unwired: 1 in]
        n129 = local read "# NCS Buffer"() -> (w372:i32)
        n130 = Not Equal?(x=w372, y=0) -> (x != y?=w373:bool)
        n131 = local write "BIO Connect"(TRUE) -> ()
        n132 = case shown="True" w373 {
          frame False {
            n133 = local write "Flush"(FALSE) -> ()
          }
          frame True {
            "Flush" <- TRUE
          }
        }
        n134 = local write "Start Acquisition"(FALSE) -> ()
        n135 = local write "Stop Acquisition"(TRUE) -> ()
        "Save" <- FALSE
        "Buffer" <- FALSE
        "Output" <- FALSE
        "Play Sound" <- FALSE
      }
      frame "Test Run" {
        w397 = "Testing"
        # "Start BIO Acquisition"
        n136 = Seconds To Date/Time(time stamp (now)=0.0) -> (date time rec=w396:T2)  [unwired: 1 in]
        n137 = local write "Start Acquisition"(TRUE) -> ()
        n138 = local write "Stop Acquisition"(FALSE) -> ()
        n139 = local write "Play Sound"(FALSE) -> ()
        n140 = local write "Save"(FALSE) -> ()
        n141 = local write "Output"(TRUE) -> ()
        n142 = local write "Flush"(FALSE) -> ()
        n143 = local write "BIO Connect"(FALSE) -> ()
        n144 = local write "Buffer"(FALSE) -> ()
      }
      frame "Training" {
        w401 = 90.0  # Routine Time
        n145 = local read "Output"() -> (w398:bool)
        n146 = Not(x=w398) -> (.not. x?=w399:bool)
        n147 = call "Elapsed Time3"("Time Target (s)"=w401, "Reset"=w399) -> ("Get Start Time (s)"=w402:dbl, "Elapsed Time (s)"=w404:dbl, "Time has Elapsed"=w400:bool)  [unwired: 10 in, 5 out]
        n148 = script code="t = [300, ...\n       310, 313, 316, 319, 322, ...\n       340, 343, 346, 349, 352, ...\n       370, 373, 376, 379, 382, 390]; % 4) Isovol\nt = t-300;\n\nevent =  [0, ...\n                6, 3, 4, 5, 0, ... % 4) Isovol\n                7, 3, 4, 5, 0, ...\n                8, 3, 4, 5, 0, 0]; \n\nfor i = 2:length(t)\n    if ((x>=t(i-1)) &&  (x<t(i)))\n        y = event(i-1);\n        yNext = event(i);\n        % dt = t(i) - t(i-1);\n        break;\n    end\nend" "Routine timing"("x"=w404) -> ("yNext"=w407:dbl, "y"=w408:dbl)  [unwired: 1 in, 1 out]
        n149 = property on="Total Routine Time" class="Slide (strict)"("Scale.Maximum"=w401) -> ()  [unwired: 2 in, 2 out]
        n150 = Seconds To Date/Time(time stamp (now)=w402) -> (date time rec=w403:T2)  [unwired: 1 in]
        n151 = case shown="False" w400 {
          frame False {
            n152 = local write "Play Sound"(TRUE) -> ()
            n153 = local write "Output"(TRUE) -> ()
            n154 = local write "Flush"(FALSE) -> ()
            n155 = local write "Save"(FALSE) -> ()
            n156 = local write "Buffer"(FALSE) -> ()
            n157 = local write "Start Acquisition"(TRUE) -> ()
            n158 = local write "Stop Acquisition"(FALSE) -> ()
            n159 = local write "BIO Connect"(FALSE) -> ()
          }
          frame True {
            n160 = local write "Play Sound"(FALSE) -> ()
            n161 = local write "Buffer"(FALSE) -> ()
            n162 = local write "Output"(FALSE) -> ()
            n163 = local write "Save"(FALSE) -> ()
            n164 = local write "Flush"(FALSE) -> ()
            n165 = local write "Start Acquisition"(FALSE) -> ()
            n166 = local write "Stop Acquisition"(TRUE) -> ()
            n167 = local write "BIO Connect"(FALSE) -> ()
            n168 = local write "Routine Selection"(enum16{"Default"}."Default") -> ()
          }
        }
        n169 = case "Next Instruction" shown="3" w407 {
          tunnel: ["Perform Normal Breathing" "Max Inhale Breath Hold" "Max Exhalation Breath Hold" "Plug Nose. Move air to chest" "Allow abdomen to relax." "Move air to abdomen." "Exhale Fully" "Inhale Fully" "Inhale Partially"] -> w406
          frame 0, Default {
          }
          frame 1 {
          }
          frame 2 {
          }
          frame 3 {
          }
          frame 4 {
          }
          frame 5 {
          }
          frame 6 {
          }
          frame 7 {
          }
          frame 8 {
          }
        }
        n170 = case "Current Instruction" shown="5" w408 {
          tunnel: ["Perform Normal Breathing" "Max Inhale Breath Hold" "Max Exhalation Breath Hold" "Plug Nose. Move air to chest" "Allow abdomen to relax." "Move air to abdomen." "Exhale Fully" "Inhale Fully" "Inhale Partially"] -> w405
          frame 0, Default {
          }
          frame 1 {
          }
          frame 2 {
          }
          frame 3 {
          }
          frame 4 {
          }
          frame 5 {
          }
          frame 6 {
          }
          frame 7 {
          }
          frame 8 {
          }
        }
      }
      frame "Routine 1" {
        w453 = 300.0  # Routine Time
        # "300"
        # "Supine Breath Monitoring"
        n171 = local read "Output"() -> (w447:bool)
        n172 = Not(x=w447) -> (.not. x?=w448:bool)
        n173 = call "Elapsed Time"("Time Target (s)"=w453, "Reset"=w448) -> ("Get Start Time (s)"=w451:dbl, "Elapsed Time (s)"=w452:dbl, "Time has Elapsed"=w449:bool)  [unwired: 10 in, 5 out]
        n174 = property on="Total Routine Time" class="Slide (strict)"("Scale.Maximum"=w453) -> ()  [unwired: 2 in, 2 out]
        n175 = Seconds To Date/Time(time stamp (now)=w451) -> (date time rec=w450:T2)  [unwired: 1 in]
        n176 = case shown="True" w449 {
          frame False {
            # "Routine Not Done. Continue buffering."
            n177 = flat-sequence {
              frame #0 {
                n178 = local write "Start Acquisition"(TRUE) -> ()
                n179 = local write "Stop Acquisition"(FALSE) -> ()
                n180 = local write "Output"(TRUE) -> ()
                n181 = local write "BIO Connect"(FALSE) -> ()
                n182 = local write "Play Sound"(TRUE) -> ()
              }
              frame #1 {
                n183 = local write "Buffer"(TRUE) -> ()
              }
            }
          }
          frame True {
            # "Routine done. Save."
            n184 = flat-sequence {
              frame #0 {
                n185 = local write "Buffer"(FALSE) -> ()
              }
              frame #1 {
                n186 = local write "Start Acquisition"(FALSE) -> ()
                n187 = local write "Stop Acquisition"(TRUE) -> ()
                n188 = local write "Output"(FALSE) -> ()
              }
              frame #2 {
                n189 = local write "Save"(TRUE) -> ()
              }
              frame #3 {
                n190 = Wait (ms)(milliseconds to wait=500) -> ()  [unwired: 1 out]
              }
              frame #4 {
                n191 = local write "Flush"(TRUE) -> ()
              }
              frame #5 {
                n192 = local write "Flush"(FALSE) -> ()
                n193 = local write "Save"(FALSE) -> ()
              }
              frame #6 {
                n194 = local write "Routine Selection"(enum16{"Default"}."Default") -> ()
                n195 = local write "Play Sound"(FALSE) -> ()
              }
            }
          }
        }
      }
      frame "Routine 2" {
        w480 = 180.0  # Routine Time
        # "Seated Breath Monitoring"
        n196 = local read "Output"() -> (w476:bool)
        n197 = Not(x=w476) -> (.not. x?=w475:bool)
        n198 = call "Elapsed Time2"("Time Target (s)"=w480, "Reset"=w475) -> ("Get Start Time (s)"=w478:dbl, "Elapsed Time (s)"=w474:dbl, "Time has Elapsed"=w477:bool)  [unwired: 10 in, 5 out]
        n199 = property on="Total Routine Time" class="Slide (strict)"("Scale.Maximum"=w480) -> ()  [unwired: 2 in, 2 out]
        n200 = Seconds To Date/Time(time stamp (now)=w478) -> (date time rec=w479:T2)  [unwired: 1 in]
        n201 = case shown="True" w477 {
          frame False {
            # "Routine Not Done. Continue buffering."
            n202 = flat-sequence {
              frame #0 {
                n203 = local write "Play Sound"(TRUE) -> ()
                n204 = local write "Start Acquisition"(TRUE) -> ()
                n205 = local write "Output"(TRUE) -> ()
                n206 = local write "Stop Acquisition"(FALSE) -> ()
                n207 = local write "BIO Connect"(FALSE) -> ()
              }
              frame #1 {
                n208 = local write "Buffer"(TRUE) -> ()
              }
            }
          }
          frame True {
            # "Routine done. Save."
            n209 = flat-sequence {
              frame #0 {
                n210 = local write "Buffer"(FALSE) -> ()
              }
              frame #1 {
                n211 = local write "Output"(FALSE) -> ()
                n212 = local write "Start Acquisition"(FALSE) -> ()
                n213 = local write "Stop Acquisition"(TRUE) -> ()
              }
              frame #2 {
                n214 = local write "Save"(TRUE) -> ()
              }
              frame #3 {
                n215 = Wait (ms)(milliseconds to wait=500) -> ()  [unwired: 1 out]
              }
              frame #4 {
                n216 = local write "Flush"(TRUE) -> ()
              }
              frame #5 {
                n217 = local write "Flush"(FALSE) -> ()
                n218 = local write "Save"(FALSE) -> ()
              }
              frame #6 {
                n219 = local write "Routine Selection"(enum16{"Default"}."Default") -> ()
                n220 = local write "Play Sound"(FALSE) -> ()
              }
            }
          }
        }
      }
      frame "Routine 3" {
        w506 = 300.0  # Routine Time
        # "Supine Heart Monitoring"
        # "180"
        n221 = local read "Output"() -> (w501:bool)
        n222 = Not(x=w501) -> (.not. x?=w502:bool)
        n223 = call "Elapsed Time4"("Time Target (s)"=w506, "Reset"=w502) -> ("Get Start Time (s)"=w504:dbl, "Elapsed Time (s)"=w507:dbl, "Time has Elapsed"=w503:bool)  [unwired: 10 in, 5 out]
        n224 = property on="Total Routine Time" class="Slide (strict)"("Scale.Maximum"=w506) -> ()  [unwired: 2 in, 2 out]
        n225 = Seconds To Date/Time(time stamp (now)=w504) -> (date time rec=w505:T2)  [unwired: 1 in]
        n226 = case shown="True" w503 {
          frame False {
            # "Routine Not Done. Continue buffering."
            n227 = flat-sequence {
              frame #0 {
                w510 = FALSE
                w509 = TRUE
                n228 = local write "Stop Acquisition"(w510) -> ()
                n229 = local write "BIO Connect"(w510) -> ()
                n230 = local write "Play Sound"(w509) -> ()
                n231 = local write "Output"(w509) -> ()
                n232 = local write "Start Acquisition"(w509) -> ()
              }
              frame #1 {
                n233 = local write "Buffer"(TRUE) -> ()
              }
            }
          }
          frame True {
            # "Routine done. Save."
            n234 = flat-sequence {
              frame #0 {
                n235 = local write "Buffer"(FALSE) -> ()
              }
              frame #1 {
                n236 = local write "Play Sound"(FALSE) -> ()
                n237 = local write "Output"(FALSE) -> ()
                n238 = local write "Start Acquisition"(FALSE) -> ()
                n239 = local write "Stop Acquisition"(TRUE) -> ()
              }
              frame #2 {
                n240 = local write "Save"(TRUE) -> ()
              }
              frame #3 {
                n241 = Wait (ms)(milliseconds to wait=500) -> ()  [unwired: 1 out]
              }
              frame #4 {
                n242 = local write "Flush"(TRUE) -> ()
              }
              frame #5 {
                n243 = local write "Flush"(FALSE) -> ()
                n244 = local write "Save"(FALSE) -> ()
              }
              frame #6 {
                n245 = local write "Routine Selection"(enum16{"Default"}."Default") -> ()
              }
            }
          }
        }
      }
      frame "Routine 4" {
        w531 = 180.0  # Routine Time
        # "Seated Heart Monitoring"
        # "300"
        n246 = local read "Output"() -> (w526:bool)
        n247 = Not(x=w526) -> (.not. x?=w527:bool)
        n248 = call "Elapsed Time5"("Time Target (s)"=w531, "Reset"=w527) -> ("Get Start Time (s)"=w529:dbl, "Elapsed Time (s)"=w525:dbl, "Time has Elapsed"=w528:bool)  [unwired: 10 in, 5 out]
        n249 = property on="Total Routine Time" class="Slide (strict)"("Scale.Maximum"=w531) -> ()  [unwired: 2 in, 2 out]
        n250 = Seconds To Date/Time(time stamp (now)=w529) -> (date time rec=w530:T2)  [unwired: 1 in]
        n251 = case shown="False" w528 {
          frame False {
            # "Routine Not Done. Continue buffering."
            n252 = flat-sequence {
              frame #0 {
                w534 = FALSE
                w533 = TRUE
                n253 = local write "Play Sound"(w533) -> ()
                n254 = local write "Stop Acquisition"(w534) -> ()
                n255 = local write "Output"(w533) -> ()
                n256 = local write "Start Acquisition"(w533) -> ()
                n257 = local write "BIO Connect"(w534) -> ()
              }
              frame #1 {
                n258 = local write "Buffer"(TRUE) -> ()
              }
            }
          }
          frame True {
            # "Routine done. Save."
            n259 = flat-sequence {
              frame #0 {
                n260 = local write "Buffer"(FALSE) -> ()
              }
              frame #1 {
                w537 = FALSE
                n261 = local write "Play Sound"(w537) -> ()
                n262 = local write "Output"(w537) -> ()
                n263 = local write "Start Acquisition"(w537) -> ()
                n264 = local write "Stop Acquisition"(TRUE) -> ()
              }
              frame #2 {
                n265 = local write "Save"(TRUE) -> ()
              }
              frame #3 {
                n266 = Wait (ms)(milliseconds to wait=500) -> ()  [unwired: 1 out]
              }
              frame #4 {
                n267 = local write "Flush"(TRUE) -> ()
              }
              frame #5 {
                n268 = local write "Flush"(FALSE) -> ()
                n269 = local write "Save"(FALSE) -> ()
              }
              frame #6 {
                n270 = local write "Routine Selection"(enum16{"Default"}."Default") -> ()
              }
            }
          }
        }
      }
      frame "Routine 5a" {
        w550 = 300.0  # Routine Time
        # "Relaxation"
        # "180"
        n271 = local read "Output"() -> (w547:bool)
        n272 = Not(x=w547) -> (.not. x?=w548:bool)
        n273 = call "Elapsed Time7"("Time Target (s)"=w550, "Reset"=w548) -> ("Get Start Time (s)"=w552:dbl, "Elapsed Time (s)"=w551:dbl, "Time has Elapsed"=w549:bool)  [unwired: 10 in, 5 out]
        n274 = property on="Total Routine Time" class="Slide (strict)"("Scale.Maximum"=w550) -> ()  [unwired: 2 in, 2 out]
        n275 = Seconds To Date/Time(time stamp (now)=w552) -> (date time rec=w554:T2)  [unwired: 1 in]
        n276 = case shown="False" w549 {
          frame False {
            n277 = flat-sequence {
              frame #0 {
                w555 = FALSE
                w556 = TRUE
                n278 = local write "Output"(w556) -> ()
                n279 = local write "Start Acquisition"(w556) -> ()
                n280 = local write "Play Sound"(w556) -> ()
                n281 = local write "Stop Acquisition"(w555) -> ()
                n282 = local write "BIO Connect"(w555) -> ()
              }
              frame #1 {
                n283 = local write "Buffer"(TRUE) -> ()
              }
            }
          }
          frame True {
            # "Routine done. Save."
            n284 = flat-sequence {
              frame #0 {
                n285 = local write "Buffer"(FALSE) -> ()
              }
              frame #1 {
                w560 = FALSE
                n286 = local write "Stop Acquisition"(TRUE) -> ()
                n287 = local write "Output"(w560) -> ()
                n288 = local write "Start Acquisition"(w560) -> ()
                n289 = local write "Play Sound"(w560) -> ()
              }
              frame #2 {
                n290 = local write "Save"(TRUE) -> ()
              }
              frame #3 {
                n291 = Wait (ms)(milliseconds to wait=500) -> ()  [unwired: 1 out]
              }
              frame #4 {
                n292 = local write "Flush"(TRUE) -> ()
              }
              frame #5 {
                n293 = local write "Flush"(FALSE) -> ()
                n294 = local write "Save"(FALSE) -> ()
              }
              frame #6 {
                n295 = local write "Routine Selection"(enum16{"Default"}."Default") -> ()
              }
            }
          }
        }
      }
      frame "Routine 5b" {
        w575 = 300.0  # Routine Time
        # "Attention"
        n296 = local read "Output"() -> (w570:bool)
        n297 = Not(x=w570) -> (.not. x?=w571:bool)
        n298 = call "Elapsed Time6"("Time Target (s)"=w575, "Reset"=w571) -> ("Get Start Time (s)"=w574:dbl, "Elapsed Time (s)"=w569:dbl, "Time has Elapsed"=w572:bool)  [unwired: 10 in, 5 out]
        n299 = property on="Total Routine Time" class="Slide (strict)"("Scale.Maximum"=w575) -> ()  [unwired: 2 in, 2 out]
        n300 = Seconds To Date/Time(time stamp (now)=w574) -> (date time rec=w573:T2)  [unwired: 1 in]
        n301 = case shown="False" w572 {
          frame False {
            # "Routine Not Done. Continue buffering."
            n302 = flat-sequence {
              tunnel: "OpenHTML" -> [w580]
              frame #0 {
                w579 = FALSE
                w578 = TRUE
                n303 = case shown="True" w580 {
                  frame False {
                  }
                  frame True {
                    n304 = local write "OpenHTML"(FALSE) -> ()
                    n305 = call-poly <vilib>:"Open URL in Default Browser.vi"("URL"="\"C:\\Users\\tbc38\\Documents\\AttentionTest\\mackworth\\vigilanceTest.html\"") -> ()  [unwired: 5 in, 2 out]
                  }
                }
                n306 = local write "Stop Acquisition"(w579) -> ()
                n307 = local write "Play Sound"(w578) -> ()
                n308 = local write "Output"(w578) -> ()
                n309 = local write "Start Acquisition"(w578) -> ()
                n310 = local write "BIO Connect"(w579) -> ()
              }
              frame #1 {
                n311 = local write "Buffer"(TRUE) -> ()
              }
            }
          }
          frame True {
            # "Routine done. Save."
            n312 = flat-sequence {
              frame #0 {
                n313 = local write "Buffer"(FALSE) -> ()
              }
              frame #1 {
                w585 = FALSE
                n314 = local write "Play Sound"(w585) -> ()
                n315 = local write "Output"(w585) -> ()
                n316 = local write "Start Acquisition"(w585) -> ()
                n317 = local write "Stop Acquisition"(TRUE) -> ()
              }
              frame #2 {
                n318 = local write "Save"(TRUE) -> ()
              }
              frame #3 {
                n319 = Wait (ms)(milliseconds to wait=500) -> ()  [unwired: 1 out]
              }
              frame #4 {
                n320 = local write "Flush"(TRUE) -> ()
              }
              frame #5 {
                n321 = local write "Save"(FALSE) -> ()
                n322 = local write "Flush"(FALSE) -> ()
              }
              frame #6 {
                n323 = local write "Routine Selection"(enum16{"Default"}."Default") -> ()
              }
            }
          }
        }
      }
    }
    "Current Routine" <- w368
    "Current Instruction" <- w362
    "Next Instruction" <- w365
    "Total Routine Time" <- w363
    "Elapsed Time" <- w364
    "Start Time" <- w361
  }
  n324 = To Unsigned Long Integer(number=w3) -> (unsigned 32bit integer=w17:u32)
  n325 = Initialize Array(0.0, w4, w17) -> (w19:dbl[][])
  n326 = property class="niUSRP"(reference=w127, error in=w128, "Carrier Frequency"="Ch3&4 carrier frequency [Hz] 2", "Bandwidth"=5000000.0 ("Configuration:Bandwidth")) -> (reference out=w98:refnum<k15>, error out=w97:errorcluster)
  n327 = Obtain Queue(max queue size (-1, unlimited)=-1, name (unnamed)="BIOPAC View", element data type=w19) -> (queue out=w10:refnum<queue>)  [unwired: 2 in, 2 out]
  n328 = property class="niUSRP"(reference=w193, error in=w194, "Carrier Frequency"="Ch1&2 carrier frequency [Hz]", "Bandwidth"=5000000.0 ("Configuration:Bandwidth")) -> (reference out=w164:refnum<k15>, error out=w163:errorcluster)
  n329 = while {
    tunnel: w10 -> [w611]
    shift-right: [w605] -> _
    shift-left: dbl[] [] -> [w606]
    shift-right: [w603] -> _
    shift-left: dbl[] [] -> [w604]
    shift-right: [w602] -> _
    shift-left: dbl[] [] -> [w601]
    shift-right: [w599] -> _
    shift-left: dbl[] [] -> [w600]
    stop <- FALSE stop-if-true
    # "SHOW/VIEWING"
    n330 = local read "ACQ ms"() -> (w594:dbl)
    n331 = local read "Receiving"() -> (w593:bool)
    n332 = Get Queue Status(queue=w611) -> (# elements in queue=w609:i32)  [unwired: 2 in, 7 out]
    "# BIOViewQ2" <- w609
    n333 = Wait (ms)(milliseconds to wait=w594) -> ()  [unwired: 1 out]
    n334 = And(x="Show BIO", y=w593) -> (x .and. y?=w607:bool)
    n335 = case shown="True" w607 {
      tunnel: w611 -> [_ w626]
      tunnel: w609 -> [_ w625]
      tunnel: w606 -> [_ w623]
      tunnel: [w612 w622] -> w605
      tunnel: w604 -> [_ w620]
      tunnel: [w612 w619] -> w603
      tunnel: [w612 w618] -> w602
      tunnel: w601 -> [_ w616]
      tunnel: [w612 w615] -> w599
      tunnel: w600 -> [_ w613]
      frame False {
        w612 = dbl[] []
      }
      frame True {
        n336 = for {
          N: w625 -> [_]
          tunnel: [w635] -> w621 mode=concatenating
          tunnel: [w632] -> w617 mode=concatenating
          tunnel: [w631] -> w614 mode=concatenating
          tunnel: w626 -> [w628]
          tunnel: [w627] -> w624 mode=concatenating
          n337 = Dequeue Element(queue=w628) -> (element=w629:dbl[][])  [unwired: 2 in, 3 out]
          n338 = Index Array(array=w629, index (row)=0) -> (element=w631:dbl[])  [unwired: 1 in]
          n339 = Index Array(array=w629, index (row)=1) -> (element=w632:dbl[])  [unwired: 1 in]
          n340 = Index Array(array=w629, index (row)=2) -> (element=w635:dbl[])  [unwired: 1 in]
          n341 = Index Array(array=w629, index (row)=3) -> (element=w627:dbl[])  [unwired: 1 in]
        }
        n342 = Build Array (concatenate)(w613, w614) -> (w615:dbl[])
        n343 = Build Array (concatenate)(w616, w617) -> (w618:dbl[])
        n344 = Build Array (concatenate)(w620, w621) -> (w619:dbl[])
        n345 = Build Array (concatenate)(w623, w624) -> (w622:dbl[])
      }
    }
    "Array 1 View" <- w599
    "Array 2 View" <- w602
    "Array 3 View" <- w603
    "Array 4 View" <- w605
    n346 = local read "# ACQ cycles"() -> (w595:i32)
    n347 = Array Size(array=w599) -> (size(s)=w598:i32)
    "View Array Size" <- w598
    n348 = Divide(x=w598, y=w594) -> (x/y=w597:dbl)
    "# Elements in Array" <- w597
    n349 = Subtract(x=w595, y=w597) -> (x-y=→"ACQ -# Elements":dbl)
  }
  n350 = property class="niUSRP"(reference=w98, error in=w97, "Active Channel"="0", "Gain"="Rx2 Gain 1", "Active Antenna"=w85) -> (reference out=w102:refnum<k15>, error out=w101:errorcluster)
  n351 = property class="niUSRP" props=["Active Channel", "Gain", "Active Antenna", "Bandwidth"](reference=w164, error in=w163, "Active Channel"="0", "Gain"="Rx1 Gain 1", "Active Antenna"=w86) -> (reference out=w168:refnum<k15>, error out=w167:errorcluster)  [unwired: 1 out]
  n352 = To Unsigned Long Integer(number=w3) -> (unsigned 32bit integer=w6:u32)
  n353 = Initialize Array(0.0, w4, w6) -> (w8:dbl[][])
  n354 = Obtain Queue(max queue size (-1, unlimited)=-1, name (unnamed)="BIOPAC Buffer", element data type=w8) -> (queue out=w2:refnum<queue>)  [unwired: 2 in, 2 out]
  n355 = while {
    tunnel: w10 -> [w637]
    tunnel: w2 -> [w639]
    stop <- FALSE stop-if-true
    # "START ACQUISITION"
    n356 = local read "Connected"() -> (w644:bool)
    n357 = local read "Receiving"() -> (w642:bool)
    n358 = Not(x=w642) -> (.not. x?=w643:bool)
    n359 = And(x=w644, y=w643) -> (x .and. y?=w645:bool)
    n360 = And(x="Start Acquisition", y=w645) -> (x .and. y?=w646:bool)
    n361 = case shown="True" w646 {
      tunnel: w637 -> [_ w651]
      tunnel: w639 -> [_ w650]
      frame False {
      }
      frame True {
        n362 = flat-sequence {
          tunnel: [w656] -> w649
          tunnel: w649 -> [w660]
          tunnel: [w660] -> w648
          tunnel: w648 -> [w662]
          tunnel: [w662] -> w652
          tunnel: w652 -> [w665]
          tunnel: w651 -> [w664]
          tunnel: w650 -> [w663]
          frame #0 {
            n363 = dll-call lib="C:/Program Files (x86)/BIOPAC Systems, Inc/BIOPAC Hardware API 2.2 Education/x64/mpdev.dll" fn="startMPAcqDaemon" label="start Acq Daemon"() -> ()  [unwired: 4 in, 2 out]
            n364 = local write "Start Acquisition"(FALSE) -> ()
            n365 = local write "Stop Acquisition"(FALSE) -> ()
            n366 = local write "Receiving"(TRUE) -> ()
          }
          frame #1 {
            w657 = u32 1  # MPSUCCESS
            n367 = dll-call lib="C:/Program Files (x86)/BIOPAC Systems, Inc/BIOPAC Hardware API 2.2 Education/x64/mpdev.dll" fn="startAcquisition" label="start Acquisition"() -> ("return type"=w658:u32)  [unwired: 3 in, 2 out]
            n368 = Equal?(x=w658, y=w657) -> (x = y?=w656:bool)
          }
          frame #2 {
            n369 = local write "Acq Started"(TRUE) -> ()
          }
          frame #3 {
            n370 = local read "ACQ ms"() -> (w661:dbl)
            n371 = Wait (ms)(milliseconds to wait=w661) -> ()  [unwired: 1 out]
          }
          frame #4 {
            n372 = local read "Sample Rate"() -> (w670:dbl)
            n373 = local read "# Channels"() -> (w668:dbl)
            n374 = local read "ACQ ms"() -> (w669:dbl)
            n375 = Reciprocal(x=w670) -> (1/x=w673:dbl)
            n376 = Multiply(x=w673, y=w669) -> (x*y=w671:dbl)
            n377 = Multiply(x=w671, y=w668) -> (x*y=w666:dbl)
            "Receive Total Size" <- w666
            n378 = Initialize Array(0.0, w666) -> (w667:dbl[])
            n379 = case shown="True" w665 {
              tunnel: w667 -> [_ w678]
              tunnel: w666 -> [_ w677]
              tunnel: w664 -> [_ w676]
              tunnel: w663 -> [_ w674]
              frame False {
              }
              frame True {
                n380 = while {
                  tunnel: w678 -> [w704]
                  tunnel: w677 -> [w703]
                  tunnel: w676 -> [w679]
                  shift-right: [w690] -> _
                  shift-left: 0 -> [w691]
                  tunnel: w674 -> [w683]
                  stop <- w686 stop-if-true
                  w701 = u32 1  # MPSUCCESS
                  n381 = Add(x=w691, y=1) -> (x+y=w690:i32)
                  "# ACQ cycles" <- w690
                  n382 = dll-call lib="C:/Program Files (x86)/BIOPAC Systems, Inc/BIOPAC Hardware API 2.2 Education/x64/mpdev.dll" fn="receiveMPData"("value"=w704, "bytetoread"=w703, "bytesread"=0) -> ("return type"=w702:i32, "value"=w696:dbl[], "bytetoread"=→"Bytes To Read":u32, "bytesread"=→"Bytes Read":i32)  [unwired: 3 in, 2 out]
                  n383 = Decimate 1D Array(w696) -> (w697:dbl[], w698:dbl[], w699:dbl[], w695:dbl[])
                  n384 = Equal?(x=w702, y=w701) -> (x = y?=w685:bool)
                  n385 = Build Array(w697, w698, w699, w695) -> (w680:dbl[][])
                  n386 = local read "Show BIO"() -> (w681:bool)
                  n387 = local write "Receive Success"(w685) -> ()
                  n388 = case shown="True" w681 {
                    tunnel: w680 -> [_ w706]
                    tunnel: w679 -> [_ w705]
                    frame False {
                    }
                    frame True {
                      n389 = Enqueue Element(queue=w705, element=w706) -> ()  [unwired: 2 in, 3 out]
                    }
                  }
                  n390 = local read "Buffer"() -> (w684:bool)
                  n391 = case shown="True" w684 {
                    tunnel: w680 -> [_ w708]
                    tunnel: w683 -> [_ w707]
                    frame False {
                    }
                    frame True {
                      n392 = Enqueue Element(queue=w707, element=w708) -> ()  [unwired: 2 in, 3 out]
                    }
                  }
                  n393 = Get Queue Status(queue=w683) -> (# elements in queue=w682:i32)  [unwired: 2 in, 7 out]
                  n394 = local write "# BIO Buffer"(w682) -> ()
                  n395 = local read "Stop Acquisition"() -> (w686:bool)
                  n396 = local read "ACQ ms"() -> (w687:dbl)
                  n397 = Subtract(x=w687, y=0.0) -> (x-y=w694:dbl)
                  n398 = Wait (ms)(milliseconds to wait=w694) -> ()  [unwired: 1 out]
                }
              }
            }
          }
          frame #5 {
            n399 = local write "Receiving"(FALSE) -> ()
            n400 = local write "Acq Started"(FALSE) -> ()
          }
        }
      }
    }
    n401 = Get Queue Status(queue=w637) -> (# elements in queue=→"# BIO View Q":i32)  [unwired: 2 in, 7 out]
    n402 = Get Queue Status(queue=w639) -> (# elements in queue=→"# BIO Buffer":i32)  [unwired: 2 in, 7 out]
  }
  n403 = property class="niUSRP"(reference=w102, error in=w101, "Active Channel"="1", "Gain"="Rx2 Gain 2", "Active Antenna"=w85) -> (reference out=w130:refnum<k15>, error out=w129:errorcluster)
  n404 = call <instrlib>:"niUSRP Open Tx Session.vi"("device names"=w150, "error in (no error)"=w129) -> ("session handle out"=w137:refnum<k15>, "error out"=w136:errorcluster)  [unwired: 12 in]
  n405 = property class="niUSRP"(reference=w137, error in=w136, "Enabled Channels"="0,1" ("Configuration:Enabled Channels")) -> (reference out=w125:refnum<k15>, error out=w124:errorcluster)
  n406 = property class="niUSRP"(reference=w125, error in=w124, "IQ Rate"="Tx IQ Rate 2") -> (reference out=w119:refnum<k15>, error out=w120:errorcluster, "IQ Rate"=w118:dbl)
  n407 = property class="niUSRP" props=["Model", "Reference Frequency Source", "Timebase Clock Source"](reference=w119, error in=w120, "Reference Frequency Source"="RefIn" ("Clocking and Synchronization:Reference Frequency Source"), "Timebase Clock Source"="PpsIn" ("Clocking and Synchronization:Timebase Clock Source")) -> (reference out=w121:refnum<k15>, error out=w122:errorcluster)  [unwired: 1 out]
  n408 = property class="niUSRP"(reference=w121, error in=w122, "Carrier Frequency"="Ch3&4 carrier frequency [Hz] 2") -> (reference out=w92:refnum<k15>, error out=w91:errorcluster)
  n409 = property class="niUSRP"(reference=w92, error in=w91, "Active Channel"="0", "Gain"="Tx2 Gain 1", "Active Antenna"=w114) -> (reference out=w96:refnum<k15>, error out=w95:errorcluster)
  n410 = property class="niUSRP"(reference=w96, error in=w95, "Active Channel"="1", "Gain"="Tx2 Gain 2", "Active Antenna"=w114) -> (reference out=w116:refnum<k15>, error out=w117:errorcluster)
  n411 = property class="niUSRP"(reference=w168, error in=w167, "Active Channel"="1", "Gain"="Rx1 Gain 2", "Active Antenna"=w86) -> (reference out=w196:refnum<k15>, error out=w195:errorcluster)
  n412 = call <instrlib>:"niUSRP Open Tx Session.vi"("device names"=w216, "error in (no error)"=w195) -> ("session handle out"=w203:refnum<k15>, "error out"=w202:errorcluster)  [unwired: 12 in]
  n413 = property class="niUSRP"(reference=w203, error in=w202, "Enabled Channels"="0,1" ("Configuration:Enabled Channels")) -> (reference out=w191:refnum<k15>, error out=w190:errorcluster)
  n414 = property class="niUSRP"(reference=w191, error in=w190, "IQ Rate"="Tx IQ Rate 1") -> (reference out=w185:refnum<k15>, error out=w186:errorcluster, "IQ Rate"=w184:dbl)
  n415 = property class="niUSRP" props=["Model", "Reference Frequency Source", "Timebase Clock Source"](reference=w185, error in=w186, "Reference Frequency Source"="RefIn" ("Clocking and Synchronization:Reference Frequency Source"), "Timebase Clock Source"="PpsIn" ("Clocking and Synchronization:Timebase Clock Source")) -> (reference out=w187:refnum<k15>, error out=w188:errorcluster)  [unwired: 1 out]
  n416 = property class="niUSRP"(reference=w187, error in=w188, "Carrier Frequency"="Ch1&2 carrier frequency [Hz]") -> (reference out=w158:refnum<k15>, error out=w157:errorcluster)
  n417 = property class="niUSRP"(reference=w158, error in=w157, "Active Channel"="0", "Gain"="Tx1 Gain 1", "Active Antenna"=w180) -> (reference out=w162:refnum<k15>, error out=w161:errorcluster)
  n418 = property class="niUSRP"(reference=w162, error in=w161, "Active Channel"="1", "Gain"="Tx1 Gain 2", "Active Antenna"=w180) -> (reference out=w182:refnum<k15>, error out=w183:errorcluster)
  n419 = while {
    stop <- FALSE stop-if-true
    # "DISCONNECT"
    n420 = Wait (ms)(milliseconds to wait=500) -> ()  [unwired: 1 out]
    n421 = case shown="True" "Disconnect" {
      frame False {
      }
      frame True {
        w714 = FALSE
        n422 = dll-call lib="C:/Program Files (x86)/BIOPAC Systems, Inc/BIOPAC Hardware API 2.2 Education/x64/mpdev.dll" fn="disconnectMPDev" label="disconnect"() -> ()  [unwired: 4 in, 2 out]
        n423 = local write "Disconnect"(w714) -> ()
        n424 = local write "Disconnected"(TRUE) -> ()
        n425 = local write "Connected"(w714) -> ()
      }
    }
  }
  n426 = while {
    stop <- FALSE stop-if-true
    n427 = local read "Output"() -> (w717:bool)
    n428 = Wait (ms)(milliseconds to wait=10.0) -> ()  [unwired: 1 out]
    n429 = case shown="True" w717 {
      tunnel: [w723 "Channel 1 Tone Amplitude"] -> w721
      tunnel: [w723 "Channel 2 Tone Amplitude"] -> w720
      tunnel: [w723 "Channel 3 Tone Amplitude"] -> w719
      tunnel: [w723 "Channel 4 Tone Amplitude"] -> w718
      frame False {
        w723 = 0.0 ("Channel 1\nTone Amplitude")
      }
      frame True {
      }
    }
    "Ch1 Amplitude" <- w721
    "Ch2 Amplitude" <- w720
    "Ch3 Amplitude" <- w719
    "Ch4 Amplitude" <- w718
  }
  n430 = call <instrlib>:"niUSRP Commit.vi"("session handle"=w116, "error in (no error)"=w117) -> ("session handle out"=w152:refnum<k15>, "error out"=w153:errorcluster)  [unwired: 12 in]
  n431 = call <instrlib>:"niUSRP Commit.vi"("session handle"=w182, "error in (no error)"=w183) -> ("session handle out"=w218:refnum<k15>, "error out"=w219:errorcluster)  [unwired: 12 in]
  n432 = Merge Errors(w129, w153) -> (w144:errorcluster)
  n433 = Merge Errors(w195, w219) -> (w210:errorcluster)
  n434 = call <instrlib>:"niUSRP Set Time.vi"("session handle"=w130, "apply timestamp"=w142, "timestamp"=T4 {"whole seconds"=0, "fractional seconds"=0.0}, "error in (no error)"=w144) -> ("session handle out"=w146:refnum<k15>, "error out"=w145:errorcluster)  [unwired: 10 in]
  n435 = call <instrlib>:"niUSRP Initiate.vi"("session handle"=w146, "error in (no error)"=w145) -> ("session handle out"=w156:refnum<k15>, "error out"=w84:errorcluster)  [unwired: 12 in]
  n436 = while {
    tunnel: w118 -> [w738]
    tunnel: w84 -> [w733]
    stop <- FALSE stop-if-true
    # "Generate I and Q waveforms."
    n437 = Bundle By Name(cluster=cluster{"Fs":dbl, "#s":dbl} {"Fs"=1000.0, "#s"=1000.0} ("sampling info"), "Fs"=w738, "#s"="Waveform Size 2") -> (w739:cluster{"Fs":dbl, "#s":dbl})
    n438 = Wait (ms)(milliseconds to wait=u32 500) -> ()  [unwired: 1 out]
    n439 = local read "Ch3 Amplitude"() -> (w729:dbl)
    n440 = local read "Ch4 Amplitude"() -> (w728:dbl)
    n441 = call <vilib>:"Sine Waveform.vi"("sampling info"=w739, "error in (no error)"=w733, "phase"=90.0, "amplitude"=w729, "frequency"="Channel 3 Tone Frequency") -> ("error out"=w734:errorcluster, "signal out"=w752:waveform(dbl))  [unwired: 5 in]
    n442 = call <vilib>:"Sine Waveform.vi"("sampling info"=w739, "error in (no error)"=w733, "amplitude"=w729, "frequency"="Channel 3 Tone Frequency") -> ("error out"=w735:errorcluster, "signal out"=w753:waveform(dbl))  [unwired: 6 in]
    n443 = call <vilib>:"Sine Waveform.vi"("sampling info"=w739, "error in (no error)"=w733, "phase"=90.0, "amplitude"=w728, "frequency"="Channel 4 Tone Frequency") -> ("error out"=w736:errorcluster, "signal out"=w743:waveform(dbl))  [unwired: 5 in]
    n444 = call <vilib>:"Sine Waveform.vi"("sampling info"=w739, "error in (no error)"=w733, "amplitude"=w728, "frequency"="Channel 4 Tone Frequency") -> ("error out"=w737:errorcluster, "signal out"=w742:waveform(dbl))  [unwired: 6 in]
    n445 = Merge Errors(w734, w735, w736, w737) -> ()  [unwired: 1 out]
    n446 = Build Array(w752, w753, w743, w742) -> (→"Tx2 Waveform Graph":waveform(dbl)[])
    n447 = Unbundle By Name(w752) -> ("Y"=w751:dbl[])
    n448 = Unbundle By Name(w753) -> ("Y"=w750:dbl[])
    n449 = Unbundle By Name(w743) -> ("Y"=w746:dbl[])
    n450 = Unbundle By Name(w742) -> ("Y"=w745:dbl[])
    n451 = Re/Im To Complex(1:w750, 2:w751) -> (0:w741:cdb[])
    n452 = Re/Im To Complex(1:w745, 2:w746) -> (0:w740:cdb[])
    n453 = Build Array(w741, w740) -> (→"Tx2 Waveform":cdb[][])
  }
  n454 = call <instrlib>:"niUSRP Set Time.vi"("session handle"=w196, "apply timestamp"=w208, "timestamp"=T4 {"whole seconds"=0, "fractional seconds"=0.0}, "error in (no error)"=w210) -> ("session handle out"=w212:refnum<k15>, "error out"=w211:errorcluster)  [unwired: 10 in]
  n455 = call <instrlib>:"niUSRP Initiate.vi"("session handle"=w212, "error in (no error)"=w211) -> ("session handle out"=w222:refnum<k15>, "error out"=w83:errorcluster)  [unwired: 12 in]
  n456 = while {
    tunnel: w184 -> [w767]
    tunnel: w83 -> [w759]
    stop <- FALSE stop-if-true
    # "Generate I and Q waveforms."
    n457 = Wait (ms)(milliseconds to wait=u32 500) -> ()  [unwired: 1 out]
    n458 = Bundle By Name(cluster=cluster{"Fs":dbl, "#s":dbl} {"Fs"=1000.0, "#s"=1000.0} ("sampling info"), "Fs"=w767, "#s"="Waveform Size 1") -> (w768:cluster{"Fs":dbl, "#s":dbl})
    n459 = local read "Ch1 Amplitude"() -> (w758:dbl)
    n460 = local read "Ch2 Amplitude"() -> (w757:dbl)
    n461 = call <vilib>:"Sine Waveform.vi"("sampling info"=w768, "error in (no error)"=w759, "phase"=90.0, "amplitude"=w758, "frequency"="Channel 1 Tone Frequency") -> ("error out"=w763:errorcluster, "signal out"=w781:waveform(dbl))  [unwired: 5 in]
    n462 = call <vilib>:"Sine Waveform.vi"("sampling info"=w768, "error in (no error)"=w759, "amplitude"=w758, "frequency"="Channel 1 Tone Frequency") -> ("error out"=w764:errorcluster, "signal out"=w782:waveform(dbl))  [unwired: 6 in]
    n463 = call <vilib>:"Sine Waveform.vi"("sampling info"=w768, "error in (no error)"=w759, "phase"=90.0, "amplitude"=w757, "frequency"="Channel 2 Tone Frequency") -> ("error out"=w765:errorcluster, "signal out"=w772:waveform(dbl))  [unwired: 5 in]
    n464 = call <vilib>:"Sine Waveform.vi"("sampling info"=w768, "error in (no error)"=w759, "amplitude"=w757, "frequency"="Channel 2 Tone Frequency") -> ("error out"=w766:errorcluster, "signal out"=w771:waveform(dbl))  [unwired: 6 in]
    n465 = Merge Errors(w763, w764, w765, w766) -> ()  [unwired: 1 out]
    n466 = Build Array(w781, w782, w772, w771) -> (→"Tx1 Waveform Graph":waveform(dbl)[])
    n467 = Unbundle By Name(w781) -> ("Y"=w780:dbl[])
    n468 = Unbundle By Name(w782) -> ("Y"=w779:dbl[])
    n469 = Unbundle By Name(w772) -> ("Y"=w775:dbl[])
    n470 = Unbundle By Name(w771) -> ("Y"=w774:dbl[])
    n471 = Re/Im To Complex(1:w779, 2:w780) -> (0:w770:cdb[])
    n472 = Re/Im To Complex(1:w774, 2:w775) -> (0:w769:cdb[])
    n473 = Build Array(w770, w769) -> (→"Tx1 Waveform":cdb[][])
  }
  n474 = local read "Waveform Size 2"() -> (w63:dbl)
  n475 = local read "Waveform Size 1"() -> (w73:dbl)
  n476 = Initialize Array(cdb 0.0+0.0i ("element"), 2 ("dimension size"), w63) -> (w65:cdb[][])
  n477 = Obtain Queue(max queue size (-1, unlimited)=-1, name (unnamed)="Rx2Queue", element data type=w65) -> (queue out=w61:refnum<queue>)  [unwired: 2 in, 2 out]
  n478 = Initialize Array(cdb 0.0+0.0i ("element"), 2 ("dimension size"), w73) -> (w70:cdb[][])
  n479 = while {
    tunnel: w61 -> [w786]
    stop <- FALSE stop-if-true
    n480 = Wait (ms)(milliseconds to wait=u32 200) -> ()  [unwired: 1 out]
    n481 = case shown="True" "Dis2" {
      tunnel: w786 -> [_ w792]
      frame False {
        n482 = Wait (ms)(milliseconds to wait=u32 500) -> ()  [unwired: 1 out]
      }
      frame True {
        n483 = Preview Queue Element(queue=w792) -> (element=w793:cdb[][])  [unwired: 2 in, 3 out]
        n484 = for {
          tunnel: w793 -> [w799] mode=indexing
          shift-right: [w796] -> w791
          shift-left: dbl[][] [] -> [w795]
          n485 = Complex To Re/Im(x + iy=w799) -> (x=w798:dbl[], y=w797:dbl[])
          n486 = Build Array (concatenate)(w795, w798, w797) -> (w796:dbl[][])
        }
        "IQ Graph 2" <- w791
      }
    }
  }
  n487 = while {
    tunnel: w156 -> [w810]
    tunnel: w84 -> [w809]
    tunnel: [w805] -> w111
    tunnel: [w808] -> w108
    shift-right: [w800] -> _
    shift-left: w61 -> [w801]
    stop <- w804 stop-if-true
    # "Rx on both channels"
    n488 = local read "Waveform Size 2"() -> (w803:dbl)
    n489 = call-poly <instrlib>:"niUSRP Fetch Rx Data (poly).vi"("session handle"=w810, "number of samples"=w803, "error in (no error)"=w809) -> ("session handle out"=w808:refnum<k15>, "data"=w802:cdb[][], "error out"=w805:errorcluster)  [unwired: 9 in, 1 out]
    n490 = Enqueue Element(queue=w801, element=w802) -> (queue out=w800:refnum<queue>)  [unwired: 2 in, 2 out]
    n491 = Unbundle By Name(w805) -> ("status"=w807:bool)
    n492 = Or(x=w807, y="Stop 2") -> (x .or. y?=w804:bool)
  }
  n493 = Obtain Queue(max queue size (-1, unlimited)=-1, name (unnamed)="Rx1Queue", element data type=w70) -> (queue out=w62:refnum<queue>)  [unwired: 2 in, 2 out]
  n494 = while {
    tunnel: w152 -> [w818]
    tunnel: w84 -> [w817]
    tunnel: [w815] -> w113
    tunnel: [w813] -> w106
    stop <- w814 stop-if-true
    # "Tx on both channels"
    n495 = local read "Tx2 Waveform"() -> (w811:cdb[][])
    n496 = local read "Stop 2"() -> (w812:bool)
    n497 = call-poly <instrlib>:"niUSRP Write Tx Data (poly).vi"("session handle"=w818, "data"=w811, "end of data?"=w812, "error in (no error)"=w817) -> ("session handle out"=w813:refnum<k15>, "error out"=w815:errorcluster)  [unwired: 10 in]
    n498 = Unbundle By Name(w815) -> ("status"=w816:bool)
    n499 = Compound Arithmetic op=OR(w816, w812) -> (w814:bool)
  }
  n500 = while {
    tunnel: w62 -> [w820]
    stop <- FALSE stop-if-true
    n501 = Wait (ms)(milliseconds to wait=u32 200) -> ()  [unwired: 1 out]
    n502 = case shown="True" "Dis1" {
      tunnel: w820 -> [_ w824]
      frame False {
        n503 = Wait (ms)(milliseconds to wait=u32 500) -> ()  [unwired: 1 out]
      }
      frame True {
        n504 = Preview Queue Element(queue=w824) -> (element=w826:cdb[][])  [unwired: 2 in, 3 out]
        n505 = for {
          tunnel: w826 -> [w832] mode=indexing
          shift-right: [w829] -> w825
          shift-left: dbl[][] [] -> [w828]
          n506 = Complex To Re/Im(x + iy=w832) -> (x=w831:dbl[], y=w830:dbl[])
          n507 = Build Array (concatenate)(w828, w831, w830) -> (w829:dbl[][])
        }
        "IQ Graph" <- w825
      }
    }
  }
  n508 = while {
    tunnel: w222 -> [w843]
    tunnel: w83 -> [w842]
    tunnel: [w838] -> w177
    tunnel: [w841] -> w174
    shift-right: [w833] -> _
    shift-left: w62 -> [w835]
    stop <- w837 stop-if-true
    # "Rx on both channels"
    n509 = local read "Waveform Size 1"() -> (w836:dbl)
    n510 = call-poly <instrlib>:"niUSRP Fetch Rx Data (poly).vi"("session handle"=w843, "number of samples"=w836, "error in (no error)"=w842) -> ("session handle out"=w841:refnum<k15>, "data"=w834:cdb[][], "error out"=w838:errorcluster)  [unwired: 9 in, 1 out]
    n511 = Enqueue Element(queue=w835, element=w834) -> (queue out=w833:refnum<queue>)  [unwired: 2 in, 2 out]
    n512 = Unbundle By Name(w838) -> ("status"=w840:bool)
    n513 = Or(x=w840, y="Stop") -> (x .or. y?=w837:bool)
  }
  n514 = while {
    tunnel: w218 -> [w851]
    tunnel: w83 -> [w850]
    tunnel: [w848] -> w179
    tunnel: [w846] -> w172
    stop <- w847 stop-if-true
    # "Tx on both channels"
    n515 = local read "Tx1 Waveform"() -> (w844:cdb[][])
    n516 = local read "Stop"() -> (w845:bool)
    n517 = call-poly <instrlib>:"niUSRP Write Tx Data (poly).vi"("session handle"=w851, "data"=w844, "end of data?"=w845, "error in (no error)"=w850) -> ("session handle out"=w846:refnum<k15>, "error out"=w848:errorcluster)  [unwired: 10 in]
    n518 = Unbundle By Name(w848) -> ("status"=w849:bool)
    n519 = Compound Arithmetic op=OR(w849, w845) -> (w847:bool)
  }
  n520 = flat-sequence {
    tunnel: [w853] -> w112
    tunnel: w113 -> [w853]
    tunnel: [w852] -> w107
    tunnel: w106 -> [w852]
    frame #0 {
      n521 = local write "Stop 2"(TRUE ("STOP")) -> ()
    }
  }
  n522 = flat-sequence {
    tunnel: [w856] -> w178
    tunnel: w179 -> [w856]
    tunnel: [w855] -> w173
    tunnel: w172 -> [w855]
    frame #0 {
      n523 = local write "Stop"(TRUE ("STOP")) -> ()
    }
  }
  n524 = flat-sequence {
    tunnel: [w859] -> w110
    tunnel: w111 -> [w859]
    tunnel: [w858] -> w109
    tunnel: w108 -> [w858]
    frame #0 {
      n525 = local write "Stop 2"(TRUE ("STOP")) -> ()
    }
  }
  n526 = flat-sequence {
    tunnel: [w862] -> w176
    tunnel: w177 -> [w862]
    tunnel: [w861] -> w175
    tunnel: w174 -> [w861]
    frame #0 {
      n527 = local write "Stop"(TRUE ("STOP")) -> ()
    }
  }
  n528 = local read "Rx IQ Rate 1"() -> (w40:dbl)
  n529 = call <instrlib>:"niUSRP Abort.vi"("session handle"=w109, "error in (no error)"=w110) -> ("session handle out"=w149:refnum<k15>, "error out"=w148:errorcluster)  [unwired: 12 in]
  n530 = local read "Waveform Size 1"() -> (w54:dbl)
  n531 = local read "DownSamplingRatio"() -> (w53:i32)
  n532 = call <instrlib>:"niUSRP Close Session.vi"("session handle"=w149, "error in (no error)"=w148) -> ("error out"=w105:errorcluster)  [unwired: 13 in]
  n533 = call <instrlib>:"niUSRP Close Session.vi"("session handle"=w107, "error in (no error)"=w112) -> ("error out"=w104:errorcluster)  [unwired: 13 in]
  n534 = Divide(x=w40, y="DownSamplingRatio1") -> (x/y=→"Sampling Rate":dbl)
  n535 = Divide(x=2000.0, y=2.0) -> (x/y=→"BW/2":dbl)
  n536 = call <instrlib>:"niUSRP Abort.vi"("session handle"=w175, "error in (no error)"=w176) -> ("session handle out"=w215:refnum<k15>, "error out"=w214:errorcluster)  [unwired: 12 in]
  n537 = flat-sequence {
    tunnel: w105 -> [w866]
    tunnel: w104 -> [w865]
    tunnel: [w864] -> w103
    frame #0 {
      n538 = Merge Errors(w866, w865) -> (w864:errorcluster)
      n539 = local write "Stop 2"(FALSE ("STOP")) -> ()
    }
  }
  n540 = Divide(x=w54, y=w53) -> (x/y=w32:dbl)
  n541 = call <instrlib>:"niUSRP Close Session.vi"("session handle"=w215, "error in (no error)"=w214) -> ("error out"=w171:errorcluster)  [unwired: 13 in]
  n542 = call <instrlib>:"niUSRP Close Session.vi"("session handle"=w173, "error in (no error)"=w178) -> ("error out"=w170:errorcluster)  [unwired: 13 in]
  n543 = flat-sequence {
    tunnel: w171 -> [w870]
    tunnel: w170 -> [w869]
    tunnel: [w868] -> w169
    frame #0 {
      n544 = Merge Errors(w870, w869) -> (w868:errorcluster)
      n545 = local write "Stop"(FALSE ("STOP")) -> ()
    }
  }
  n546 = Initialize Array(0.0 ("element"), w33, w32) -> (w55:dbl[][])
  n547 = Initialize Array(0.0 ("element"), w33, w32) -> (w42:dbl[][])
  n548 = Obtain Queue(name (unnamed)="Buffer", element data type=w42) -> (queue out=w41:refnum<queue>)  [unwired: 3 in, 2 out]
  n549 = Obtain Queue(name (unnamed)="ChsQueue", element data type=w55) -> (queue out=w52:refnum<queue>)  [unwired: 3 in, 2 out]
  n550 = while {
    tunnel: w62 -> [w1072]
    tunnel: w61 -> [w1069]
    tunnel: w52 -> [w1029]
    tunnel: w41 -> [w1027]
    tunnel: w2 -> [w879]
    stop <- FALSE stop-if-true
    w873 = 2 ("order")
    w902 = Filter_Passband_Type."Bandpass" ("filter type")
    w932 = Filter_Passband_Type."Bandpass" ("filter type")
    w872 = Filter_Passband_Type."Bandpass" ("filter type")
    w972 = Filter_Passband_Type."Bandpass" ("filter type")
    w874 = 2 ("order")
    # "Tx4 to Rx4 QueInd_15"
    # "Tx3 to Rx4 QueInd_14"
    # "Tx2 to Rx4 QueInd_13"
    # "Tx1 to Rx4 QueInd_12"
    # "Tx4 to Rx3 QueInd_11"
    # "Tx3 to Rx3 QueInd_10"
    # "Tx2 to Rx3 QueInd_9"
    # "Tx1 to Rx3 QueInd_8"
    # "Tx1 to Rx4 QueInd_12"
    # "Tx2 to Rx4 QueInd_13"
    # "Tx2 to Rx3 QueInd_9"
    # "Tx1 to Rx3 QueInd_8"
    # "Tx4 to Rx2 QueInd_7"
    # "Tx3 to Rx2 QueInd_6"
    # "Tx4 to Rx1 QueInd_3"
    # "Tx3 to Rx1 QueInd_2"
    # "Tx4 to Rx2 QueInd_7"
    # "Tx4 to Rx4 QueInd_15"
    # "Tx3 to Rx2 QueInd_6"
    # "Tx4 to Rx3 QueInd_11"
    # "Tx2 to Rx2 QueInd_5"
    # "Tx2 to Rx2 QueInd_5"
    # "Tx1 to Rx2 QueInd_4"
    # "Tx4 to Rx1 QueInd_3"
    # "Tx3 to Rx1 QueInd_2"
    # "Tx2 to Rx1 QueInd_1"
    # "Tx1 to Rx1 QueInd_0"
    # "Tx2 to Rx1 QueInd_1"
    # "Tx3 to Rx4 QueInd_14"
    # "Tx3 to Rx3 QueInd_10"
    # "Tx1 to Rx2 QueInd_4"
    # "Tx1 to Rx1 QueInd_0"
    # "100 times"
    n551 = Dequeue Element(queue=w1072) -> (element=w1074:cdb[][])  [unwired: 2 in, 3 out]
    n552 = Get Queue Status(queue=w1072) -> (# elements in queue=→"# IQ queue Ch 1":i32)  [unwired: 2 in, 7 out]
    n553 = Get Queue Status(queue=w1069) -> (# elements in queue=→"# IQ queue Ch 2":i32)  [unwired: 2 in, 7 out]
    n554 = Dequeue Element(queue=w1069) -> (element=w1066:cdb[][])  [unwired: 2 in, 3 out]
    n555 = Index Array(array=w1074, index (row)=1) -> (element=w955:cdb[])  [unwired: 1 in]
    n556 = Index Array(array=w1074, index (row)=0) -> (element=w975:cdb[])  [unwired: 1 in]
    n557 = Index Array(array=w1066, index (row)=1) -> (element=w908:cdb[])  [unwired: 1 in]
    n558 = Index Array(array=w1066, index (row)=0) -> (element=w875:cdb[])  [unwired: 1 in]
    n559 = local read "Channel 2 Tone Frequency"() -> (w1014:dbl)
    n560 = local read "Channel 1 Tone Frequency"() -> (w1026:dbl)
    n561 = local read "Channel 3 Tone Frequency"() -> (w956:dbl)
    n562 = local read "Channel 4 Tone Frequency"() -> (w943:dbl)
    n563 = local read "Channel 4 Tone Frequency"() -> (w974:dbl)
    n564 = local read "Channel 3 Tone Frequency"() -> (w1047:dbl)
    n565 = local read "Channel 3 Tone Frequency"() -> (w985:dbl)
    n566 = local read "Channel 4 Tone Frequency"() -> (w994:dbl)
    n567 = local read "Channel 2 Tone Frequency"() -> (w1021:dbl)
    n568 = local read "Channel 2 Tone Frequency"() -> (w901:dbl)
    n569 = local read "Channel 1 Tone Frequency"() -> (w1063:dbl)
    n570 = local read "Channel 1 Tone Frequency"() -> (w914:dbl)
    n571 = local read "Rx IQ Rate 1"() -> (w976:dbl)
    n572 = local read "Channel 1 Tone Frequency"() -> (w939:dbl)
    n573 = local read "Channel 2 Tone Frequency"() -> (w919:dbl)
    n574 = local read "Channel 3 Tone Frequency"() -> (w1052:dbl)
    n575 = local read "Channel 4 Tone Frequency"() -> (w1005:dbl)
    n576 = local read "Rx IQ Rate 2"() -> (w907:dbl)
    n577 = local read "BW/2"() -> (w973:dbl)
    n578 = local read "BW/2"() -> (w946:dbl)
    n579 = local read "Rx IQ Rate 1"() -> (w954:dbl)
    n580 = local read "Rx IQ Rate 2"() -> (w922:dbl)
    n581 = local read "BW/2"() -> (w909:dbl)
    n582 = local read "BW/2"() -> (w920:dbl)
    n583 = Subtract(x=w956, y=w946) -> (x-y=w960:dbl)
    n584 = Subtract(x=w974, y=w973) -> (x-y=w978:dbl)
    n585 = Subtract(x=w1014, y=w946) -> (x-y=w1012:dbl)
    n586 = Add(x=w956, y=w946) -> (x+y=w961:dbl)
    n587 = Add(x=w943, y=w946) -> (x+y=w944:dbl)
    n588 = Subtract(x=w943, y=w946) -> (x-y=w945:dbl)
    n589 = Subtract(x=w901, y=w909) -> (x-y=w906:dbl)
    n590 = Subtract(x=w1063, y=w973) -> (x-y=w1064:dbl)
    n591 = Add(x=w974, y=w973) -> (x+y=w979:dbl)
    n592 = Add(x=w1014, y=w946) -> (x+y=w1013:dbl)
    n593 = Subtract(x=w1021, y=w973) -> (x-y=w1022:dbl)
    n594 = Subtract(x=w985, y=w973) -> (x-y=w986:dbl)
    n595 = Subtract(x=w914, y=w909) -> (x-y=w915:dbl)
    n596 = Add(x=w901, y=w909) -> (x+y=w905:dbl)
    n597 = Add(x=w1063, y=w973) -> (x+y=w1065:dbl)
    n598 = Add(x=w1021, y=w973) -> (x+y=w1023:dbl)
    n599 = Add(x=w985, y=w973) -> (x+y=w987:dbl)
    n600 = Add(x=w914, y=w909) -> (x+y=w916:dbl)
    n601 = Subtract(x=w1026, y=w946) -> (x-y=w1059:dbl)
    n602 = Add(x=w1026, y=w946) -> (x+y=w1060:dbl)
    n603 = Subtract(x=w994, y=w909) -> (x-y=w995:dbl)
    n604 = Add(x=w994, y=w909) -> (x+y=w996:dbl)
    n605 = Subtract(x=w1047, y=w909) -> (x-y=w1050:dbl)
    n606 = Add(x=w1047, y=w909) -> (x+y=w1051:dbl)
    n607 = Subtract(x=w939, y=w920) -> (x-y=w938:dbl)
    n608 = Subtract(x=w1005, y=w920) -> (x-y=w1003:dbl)
    n609 = Add(x=w939, y=w920) -> (x+y=w937:dbl)
    n610 = Add(x=w1005, y=w920) -> (x+y=w1004:dbl)
    n611 = Subtract(x=w919, y=w920) -> (x-y=w921:dbl)
    n612 = Subtract(x=w1052, y=w920) -> (x-y=w1055:dbl)
    n613 = Add(x=w919, y=w920) -> (x+y=w923:dbl)
    n614 = Add(x=w1052, y=w920) -> (x+y=w1056:dbl)
    n615 = call-poly <vilib>:"Butterworth Filter.vi"("init/cont (init:F)"=TRUE, "order"=w874, "filter type"=w972, "low cutoff freq: fl"=w978, "high cutoff freq: fh"=w979, "sampling freq: fs"=w976, "X"=w975) -> ("Filtered X"=w971:cdb[])  [unwired: 1 in, 1 out]
    n616 = call-poly <vilib>:"Butterworth Filter.vi"("init/cont (init:F)"=TRUE, "order"=w874, "filter type"=w972, "low cutoff freq: fl"=w1022, "high cutoff freq: fh"=w1023, "sampling freq: fs"=w976, "X"=w975) -> ("Filtered X"=w1020:cdb[])  [unwired: 1 in, 1 out]
    n617 = call-poly <vilib>:"Butterworth Filter.vi"("init/cont (init:F)"=TRUE, "order"=w874, "filter type"=w972, "low cutoff freq: fl"=w986, "high cutoff freq: fh"=w987, "sampling freq: fs"=w976, "X"=w975) -> ("Filtered X"=w984:cdb[])  [unwired: 1 in, 1 out]
    n618 = call-poly <vilib>:"Butterworth Filter.vi"("init/cont (init:F)"=TRUE, "order"=w874, "filter type"=w972, "low cutoff freq: fl"=w1064, "high cutoff freq: fh"=w1065, "sampling freq: fs"=w976, "X"=w975) -> ("Filtered X"=w1062:cdb[])  [unwired: 1 in, 1 out]
    n619 = call-poly <vilib>:"Butterworth Filter.vi"("init/cont (init:F)"=TRUE, "order"=w874, "filter type"=w872, "low cutoff freq: fl"=w1059, "high cutoff freq: fh"=w1060, "sampling freq: fs"=w954, "X"=w955) -> ("Filtered X"=w1058:cdb[])  [unwired: 1 in, 1 out]
    n620 = call-poly <vilib>:"Butterworth Filter.vi"("init/cont (init:F)"=TRUE, "order"=w873, "filter type"=w902, "low cutoff freq: fl"=w906, "high cutoff freq: fh"=w905, "sampling freq: fs"=w907, "X"=w908) -> ("Filtered X"=w903:cdb[])  [unwired: 1 in, 1 out]
    n621 = call-poly <vilib>:"Butterworth Filter.vi"("init/cont (init:F)"=TRUE, "order"=w874, "filter type"=w872, "low cutoff freq: fl"=w960, "high cutoff freq: fh"=w961, "sampling freq: fs"=w954, "X"=w955) -> ("Filtered X"=w959:cdb[])  [unwired: 1 in, 1 out]
    n622 = call-poly <vilib>:"Butterworth Filter.vi"("init/cont (init:F)"=TRUE, "order"=w874, "filter type"=w872, "low cutoff freq: fl"=w945, "high cutoff freq: fh"=w944, "sampling freq: fs"=w954, "X"=w955) -> ("Filtered X"=w952:cdb[])  [unwired: 1 in, 1 out]
    n623 = call-poly <vilib>:"Butterworth Filter.vi"("init/cont (init:F)"=TRUE, "order"=w873, "filter type"=w902, "low cutoff freq: fl"=w915, "high cutoff freq: fh"=w916, "sampling freq: fs"=w907, "X"=w908) -> ("Filtered X"=w918:cdb[])  [unwired: 1 in, 1 out]
    n624 = call-poly <vilib>:"Butterworth Filter.vi"("init/cont (init:F)"=TRUE, "order"=w874, "filter type"=w872, "low cutoff freq: fl"=w1012, "high cutoff freq: fh"=w1013, "sampling freq: fs"=w954, "X"=w955) -> ("Filtered X"=w1011:cdb[])  [unwired: 1 in, 1 out]
    n625 = call-poly <vilib>:"Butterworth Filter.vi"("init/cont (init:F)"=TRUE, "order"=w873, "filter type"=w902, "low cutoff freq: fl"=w995, "high cutoff freq: fh"=w996, "sampling freq: fs"=w907, "X"=w908) -> ("Filtered X"=w993:cdb[])  [unwired: 1 in, 1 out]
    n626 = call-poly <vilib>:"Butterworth Filter.vi"("init/cont (init:F)"=TRUE, "order"=w873, "filter type"=w902, "low cutoff freq: fl"=w1050, "high cutoff freq: fh"=w1051, "sampling freq: fs"=w907, "X"=w908) -> ("Filtered X"=w1049:cdb[])  [unwired: 1 in, 1 out]
    n627 = call-poly <vilib>:"Butterworth Filter.vi"("init/cont (init:F)"=TRUE, "order"=w873, "filter type"=w932, "low cutoff freq: fl"=w938, "high cutoff freq: fh"=w937, "sampling freq: fs"=w922, "X"=w875) -> ("Filtered X"=w941:cdb[])  [unwired: 1 in, 1 out]
    n628 = call-poly <vilib>:"Butterworth Filter.vi"("init/cont (init:F)"=TRUE, "order"=w873, "filter type"=w932, "low cutoff freq: fl"=w921, "high cutoff freq: fh"=w923, "sampling freq: fs"=w922, "X"=w875) -> ("Filtered X"=w931:cdb[])  [unwired: 1 in, 1 out]
    n629 = call-poly <vilib>:"Butterworth Filter.vi"("init/cont (init:F)"=TRUE, "order"=w873, "filter type"=w932, "low cutoff freq: fl"=w1003, "high cutoff freq: fh"=w1004, "sampling freq: fs"=w922, "X"=w875) -> ("Filtered X"=w1002:cdb[])  [unwired: 1 in, 1 out]
    n630 = call-poly <vilib>:"Butterworth Filter.vi"("init/cont (init:F)"=TRUE, "order"=w873, "filter type"=w932, "low cutoff freq: fl"=w1055, "high cutoff freq: fh"=w1056, "sampling freq: fs"=w922, "X"=w875) -> ("Filtered X"=w1054:cdb[])  [unwired: 1 in, 1 out]
    n631 = Complex To Polar(r * e^(i*theta)=w971) -> (r=w970:dbl[])  [unwired: 1 out]
    n632 = Complex To Polar(r * e^(i*theta)=w984) -> (r=w982:dbl[])  [unwired: 1 out]
    n633 = Complex To Polar(r * e^(i*theta)=w1020) -> (r=w1019:dbl[])  [unwired: 1 out]
    n634 = Complex To Polar(r * e^(i*theta)=w1062) -> (r=w1046:dbl[])  [unwired: 1 out]
    n635 = Complex To Polar(r * e^(i*theta)=w959) -> (r=w958:dbl[])  [unwired: 1 out]
    n636 = Complex To Polar(r * e^(i*theta)=w952) -> (r=w951:dbl[])  [unwired: 1 out]
    n637 = Complex To Polar(r * e^(i*theta)=w1058) -> (r=w1033:dbl[])  [unwired: 1 out]
    n638 = Complex To Polar(r * e^(i*theta)=w1011) -> (r=w1010:dbl[])  [unwired: 1 out]
    n639 = local read "DownSamplingRatio"() -> (w948:i32)
    n640 = local read "DownSamplingRatio"() -> (w965:i32)
    n641 = Complex To Polar(r * e^(i*theta)=w941) -> (r=w940:dbl[])  [unwired: 1 out]
    n642 = Complex To Polar(r * e^(i*theta)=w931) -> (r=w930:dbl[])  [unwired: 1 out]
    n643 = Complex To Polar(r * e^(i*theta)=w1054) -> (r=w1032:dbl[])  [unwired: 1 out]
    n644 = Complex To Polar(r * e^(i*theta)=w1002) -> (r=w1001:dbl[])  [unwired: 1 out]
    n645 = Complex To Polar(r * e^(i*theta)=w903) -> (r=w895:dbl[])  [unwired: 1 out]
    n646 = Complex To Polar(r * e^(i*theta)=w918) -> (r=w911:dbl[])  [unwired: 1 out]
    n647 = local read "Waveform Size 1"() -> (w968:dbl)
    n648 = Complex To Polar(r * e^(i*theta)=w1049) -> (r=w1031:dbl[])  [unwired: 1 out]
    n649 = Complex To Polar(r * e^(i*theta)=w993) -> (r=w992:dbl[])  [unwired: 1 out]
    n650 = local read "DownSamplingRatio"() -> (w897:i32)
    n651 = local read "DownSamplingRatio"() -> (w926:i32)
    n652 = local read "Waveform Size 1"() -> (w949:dbl)
    n653 = local read "Waveform Size 2"() -> (w928:dbl)
    n654 = local read "Waveform Size 2"() -> (w898:dbl)
    n655 = Divide(x=w949, y=w948) -> (x/y=w957:dbl)
    n656 = Divide(x=w949, y=w948) -> (x/y=w950:dbl)
    n657 = Divide(x=w949, y=w948) -> (x/y=w1009:dbl)
    n658 = Divide(x=w968, y=w965) -> (x/y=w969:dbl)
    n659 = Divide(x=w968, y=w965) -> (x/y=w1018:dbl)
    n660 = Divide(x=w968, y=w965) -> (x/y=w983:dbl)
    n661 = Divide(x=w968, y=w965) -> (x/y=w1045:dbl)
    n662 = Divide(x=w949, y=w948) -> (x/y=w1034:dbl)
    n663 = Divide(x=w928, y=w926) -> (x/y=w934:dbl)
    n664 = Divide(x=w898, y=w897) -> (x/y=w991:dbl)
    n665 = Divide(x=w928, y=w926) -> (x/y=w929:dbl)
    n666 = Divide(x=w928, y=w926) -> (x/y=w1000:dbl)
    n667 = Divide(x=w898, y=w897) -> (x/y=w896:dbl)
    n668 = Reshape Array(w958, w957, w948) -> (w963:dbl[][])
    n669 = Divide(x=w928, y=w926) -> (x/y=w1040:dbl)
    n670 = Reshape Array(w951, w950, w948) -> (w933:dbl[][])
    n671 = Divide(x=w898, y=w897) -> (x/y=w912:dbl)
    n672 = Divide(x=w898, y=w897) -> (x/y=w1037:dbl)
    n673 = Reshape Array(w1010, w1009, w948) -> (w1008:dbl[][])
    n674 = Reshape Array(w970, w969, w965) -> (w967:dbl[][])
    n675 = Reshape Array(w982, w983, w965) -> (w981:dbl[][])
    n676 = Reshape Array(w1046, w1045, w965) -> (w1044:dbl[][])
    n677 = Reshape Array(w1033, w1034, w948) -> (w1042:dbl[][])
    n678 = Reshape Array(w1019, w1018, w965) -> (w1017:dbl[][])
    n679 = Reshape Array(w940, w934, w926) -> (w936:dbl[][])
    n680 = Reshape Array(w992, w991, w897) -> (w990:dbl[][])
    n681 = Reshape Array(w930, w929, w926) -> (w927:dbl[][])
    n682 = Reshape Array(w1001, w1000, w926) -> (w999:dbl[][])
    n683 = Reshape Array(w895, w896, w897) -> (w900:dbl[][])
    n684 = Reshape Array(w1032, w1040, w926) -> (w1039:dbl[][])
    n685 = Reshape Array(w911, w912, w897) -> (w913:dbl[][])
    n686 = Reshape Array(w1031, w1037, w897) -> (w1036:dbl[][])
    n687 = for {
      tunnel: w1044 -> [w1115] mode=indexing
      tunnel: [w1114] -> w1043 mode=indexing
      workers-P: _ -> [_]
      n688 = Add Array Elements(numeric array=w1115) -> (sum=w1114:dbl)
    }
    n689 = for {
      tunnel: w1017 -> [w1100] mode=indexing
      tunnel: [w1099] -> w1016 mode=indexing
      workers-P: _ -> [_]
      n690 = Add Array Elements(numeric array=w1100) -> (sum=w1099:dbl)
    }
    n691 = for {
      tunnel: w981 -> [w1092] mode=indexing
      tunnel: [w1091] -> w980 mode=indexing
      workers-P: _ -> [_]
      n692 = Add Array Elements(numeric array=w1092) -> (sum=w1091:dbl)
    }
    n693 = for {
      tunnel: w967 -> [w1090] mode=indexing
      tunnel: [w1089] -> w966 mode=indexing
      workers-P: _ -> [_]
      n694 = Add Array Elements(numeric array=w1090) -> (sum=w1089:dbl)
    }
    n695 = for {
      tunnel: w963 -> [w1088] mode=indexing
      tunnel: [w1087] -> w964 mode=indexing
      workers-P: _ -> [_]
      n696 = Add Array Elements(numeric array=w1088) -> (sum=w1087:dbl)
    }
    n697 = for {
      tunnel: w1042 -> [w1113] mode=indexing
      tunnel: [w1112] -> w1041 mode=indexing
      workers-P: _ -> [_]
      n698 = Add Array Elements(numeric array=w1113) -> (sum=w1112:dbl)
    }
    n699 = for {
      tunnel: w933 -> [w1086] mode=indexing
      tunnel: [w1085] -> w947 mode=indexing
      workers-P: _ -> [_]
      n700 = Add Array Elements(numeric array=w1086) -> (sum=w1085:dbl)
    }
    n701 = for {
      tunnel: w1008 -> [w1098] mode=indexing
      tunnel: [w1097] -> w1007 mode=indexing
      workers-P: _ -> [_]
      n702 = Add Array Elements(numeric array=w1098) -> (sum=w1097:dbl)
    }
    n703 = for {
      tunnel: w936 -> [w1084] mode=indexing
      tunnel: [w1083] -> w935 mode=indexing
      workers-P: _ -> [_]
      n704 = Add Array Elements(numeric array=w1084) -> (sum=w1083:dbl)
    }
    n705 = for {
      tunnel: w927 -> [w1082] mode=indexing
      tunnel: [w1081] -> w925 mode=indexing
      workers-P: _ -> [_]
      n706 = Add Array Elements(numeric array=w1082) -> (sum=w1081:dbl)
    }
    n707 = for {
      tunnel: w999 -> [w1096] mode=indexing
      tunnel: [w1095] -> w998 mode=indexing
      workers-P: _ -> [_]
      n708 = Add Array Elements(numeric array=w1096) -> (sum=w1095:dbl)
    }
    n709 = for {
      tunnel: w900 -> [w1078] mode=indexing
      tunnel: [w1077] -> w899 mode=indexing
      workers-P: _ -> [_]
      n710 = Add Array Elements(numeric array=w1078) -> (sum=w1077:dbl)
    }
    n711 = for {
      tunnel: w1039 -> [w1111] mode=indexing
      tunnel: [w1110] -> w1038 mode=indexing
      workers-P: _ -> [_]
      n712 = Add Array Elements(numeric array=w1111) -> (sum=w1110:dbl)
    }
    n713 = for {
      tunnel: w913 -> [w1080] mode=indexing
      tunnel: [w1079] -> w910 mode=indexing
      workers-P: _ -> [_]
      n714 = Add Array Elements(numeric array=w1080) -> (sum=w1079:dbl)
    }
    n715 = for {
      tunnel: w1036 -> [w1109] mode=indexing
      tunnel: [w1108] -> w1035 mode=indexing
      workers-P: _ -> [_]
      n716 = Add Array Elements(numeric array=w1109) -> (sum=w1108:dbl)
    }
    n717 = for {
      tunnel: w990 -> [w1094] mode=indexing
      tunnel: [w1093] -> w989 mode=indexing
      workers-P: _ -> [_]
      n718 = Add Array Elements(numeric array=w1094) -> (sum=w1093:dbl)
    }
    n719 = Divide(x=w964, y=w948) -> (x/y=w889:dbl[])
    n720 = Divide(x=w947, y=w948) -> (x/y=w888:dbl[])
    n721 = Divide(x=w1007, y=w948) -> (x/y=w890:dbl[])
    n722 = Divide(x=w1043, y=w965) -> (x/y=w1030:dbl[])
    n723 = Divide(x=w1041, y=w948) -> (x/y=w891:dbl[])
    n724 = Divide(x=w1016, y=w965) -> (x/y=w894:dbl[])
    n725 = Divide(x=w980, y=w965) -> (x/y=w893:dbl[])
    n726 = Divide(x=w966, y=w965) -> (x/y=w892:dbl[])
    n727 = Divide(x=w935, y=w926) -> (x/y=w887:dbl[])
    n728 = Divide(x=w925, y=w926) -> (x/y=w886:dbl[])
    n729 = Divide(x=w1038, y=w926) -> (x/y=w885:dbl[])
    n730 = Divide(x=w998, y=w926) -> (x/y=w884:dbl[])
    n731 = Divide(x=w899, y=w897) -> (x/y=w881:dbl[])
    n732 = Divide(x=w1035, y=w897) -> (x/y=w882:dbl[])
    n733 = Divide(x=w910, y=w897) -> (x/y=w880:dbl[])
    n734 = Divide(x=w989, y=w897) -> (x/y=w883:dbl[])
    n735 = Build Array(w1030, w894, w893, w892, w891, w890, w889, w888, w887, w886, w885, w884, w880, w881, w882, w883) -> (w1028:dbl[][])
    "ChAmp" <- w1028
    n736 = local read "Acq Started"() -> (w876:bool)
    n737 = local read "Buffer"() -> (w877:bool)
    n738 = local read "Flush"() -> (w1025:bool)
    n739 = And(x=w876, y=w877) -> (x .and. y?=w878:bool)
    n740 = case shown="True" w878 {
      tunnel: w1027 -> [w1103 w1107]
      tunnel: w1028 -> [_ w1106]
      tunnel: w1025 -> [w1102 _]
      tunnel: w879 -> [w1101 _]
      frame False {
        n741 = case shown="True" w1102 {
          tunnel: w1103 -> [_ w1105]
          tunnel: w1101 -> [_ w1104]
          frame False {
          }
          frame True {
            n742 = Flush Queue(queue=w1104) -> ()  [unwired: 1 in, 3 out]
            n743 = Flush Queue(queue=w1105) -> ()  [unwired: 1 in, 3 out]
          }
        }
      }
      frame True {
        n744 = Enqueue Element(queue=w1107, element=w1106) -> ()  [unwired: 2 in, 3 out]
      }
    }
    n745 = Enqueue Element(queue=w1029, element=w1028) -> ()  [unwired: 2 in, 3 out]
  }
  n746 = local read "DownSamplingRatio"() -> (w50:i32)
  n747 = local read "Waveform Size 1"() -> (w51:dbl)
  n748 = Divide(x=w51, y=w50) -> (x/y=w37:dbl)
  n749 = Divide(x=w37, y="DownSamplingRatio 2") -> (x/y=w28:dbl)
  n750 = Multiply(x=w27, y=w28) -> (x*y=w45:dbl)
  n751 = Initialize Array(w26, w27, w28) -> (w49:dbl[][])
  n752 = Initialize Array(w26, w27, w28) -> (w48:dbl[][])
  n753 = Initialize Array(w26, w27, w28) -> (w47:dbl[][])
  n754 = Initialize Array(w26, w27, w28) -> (w46:dbl[][])
  n755 = Initialize Array(w26, w27, w28) -> (w25:dbl[][])
  n756 = Initialize Array(w26, w27, w28) -> (w24:dbl[][])
  n757 = Initialize Array(w26, w27, w28) -> (w23:dbl[][])
  n758 = Initialize Array(w26, w27, w28) -> (w22:dbl[][])
  n759 = while {
    tunnel: w27 -> [w1229]
    tunnel: w52 -> [w1222]
    shift-right: [w1219] -> _
    shift-left: w49 -> [w1201]
    tunnel: w45 -> [w1137]
    shift-right: [w1213] -> _
    shift-left: w48 -> [w1225]
    shift-right: [w1212] -> _
    shift-left: w47 -> [w1224]
    shift-right: [w1211] -> _
    shift-left: w46 -> [w1223]
    tunnel: "DownSamplingRatio 2" -> [w1152]
    tunnel: w28 -> [w1161]
    tunnel: "DownSamplingRatio 2" -> [w1185]
    shift-right: [w1133] -> _
    shift-left: w25 -> [w1147]
    shift-right: [w1132] -> _
    shift-left: w24 -> [w1139]
    shift-right: [w1131] -> _
    shift-left: w23 -> [w1142]
    shift-right: [w1130] -> _
    shift-left: w22 -> [w1149]
    stop <- FALSE stop-if-true
    # "Tx4 to Rx4 QueInd_15"
    # "Tx3 to Rx4 QueInd_14"
    # "Tx2 to Rx4 QueInd_13"
    # "Tx1 to Rx4 QueInd_12"
    # "Tx4 to Rx3 QueInd_11"
    # "Tx3 to Rx3 QueInd_10"
    # "Tx2 to Rx3 QueInd_9"
    # "Tx1 to Rx3 QueInd_8"
    # "Tx4 to Rx2 QueInd_7"
    # "Tx3 to Rx2 QueInd_6"
    # "Tx2 to Rx2 QueInd_5"
    # "Tx1 to Rx2 QueInd_4"
    # "Tx4 to Rx1 QueInd_3"
    # "Tx3 to Rx1 QueInd_2"
    # "Tx2 to Rx1 QueInd_1"
    # "Tx1 to Rx1 QueInd_0"
    n760 = local read "Sampling Rate"() -> (w1186:dbl)
    n761 = Get Queue Status(queue=w1222) -> (# elements in queue=→"# elements in view queue":i32)  [unwired: 2 in, 7 out]
    n762 = Dequeue Element(queue=w1222) -> (element=w1166:dbl[][])  [unwired: 2 in, 3 out]
    n763 = Decrement(x=w1229) -> (x-1=w1140:i32)
    n764 = Divide(x=w1186, y=w1185) -> (x/y=→"Dis Sampling Rate":dbl)
    n765 = Index Array(array=w1166, index (row)=10 ("index")) -> (element=w1165:dbl[])  [unwired: 1 in]
    n766 = Index Array(array=w1166, index (row)=11 ("index")) -> (element=w1164:dbl[])  [unwired: 1 in]
    n767 = Index Array(array=w1166, index (row)=15 ("index")) -> (element=w1163:dbl[])  [unwired: 1 in]
    n768 = Index Array(array=w1166, index (row)=14 ("index")) -> (element=w1162:dbl[])  [unwired: 1 in]
    n769 = Index Array(array=w1166, index (row)=0 ("index")) -> (element=w1199:dbl[])  [unwired: 1 in]
    n770 = Index Array(array=w1166, index (row)=1 ("index")) -> (element=w1198:dbl[])  [unwired: 1 in]
    n771 = Index Array(array=w1166, index (row)=5 ("index")) -> (element=w1197:dbl[])  [unwired: 1 in]
    n772 = Index Array(array=w1166, index (row)=4 ("index")) -> (element=w1196:dbl[])  [unwired: 1 in]
    n773 = Array Subset(array=w1142, index (row)=0 ("index"), length (row)=w1140) -> (w1141:dbl[][])  [unwired: 2 in]
    n774 = Array Subset(array=w1149, index (row)=0 ("index"), length (row)=w1140) -> (w1148:dbl[][])  [unwired: 2 in]
    n775 = Array Subset(array=w1139, index (row)=0 ("index"), length (row)=w1140) -> (w1138:dbl[][])  [unwired: 2 in]
    n776 = Array Subset(array=w1147, index (row)=0 ("index"), length (row)=w1140) -> (w1146:dbl[][])  [unwired: 2 in]
    n777 = Array Subset(array=w1201, index (row)=0 ("index"), length (row)=w1140) -> (w1220:dbl[][])  [unwired: 2 in]
    n778 = Array Subset(array=w1225, index (row)=0 ("index"), length (row)=w1140) -> (w1216:dbl[][])  [unwired: 2 in]
    n779 = Array Subset(array=w1224, index (row)=0 ("index"), length (row)=w1140) -> (w1215:dbl[][])  [unwired: 2 in]
    n780 = Array Subset(array=w1223, index (row)=0 ("index"), length (row)=w1140) -> (w1214:dbl[][])  [unwired: 2 in]
    n781 = Reshape Array(w1164, w1161, w1152) -> (w1159:dbl[][])
    n782 = Reshape Array(w1163, w1161, w1152) -> (w1158:dbl[][])
    n783 = Reshape Array(w1162, w1161, w1152) -> (w1157:dbl[][])
    n784 = Reshape Array(w1198, w1161, w1152) -> (w1193:dbl[][])
    n785 = Reshape Array(w1197, w1161, w1152) -> (w1192:dbl[][])
    n786 = Reshape Array(w1196, w1161, w1152) -> (w1191:dbl[][])
    n787 = Reshape Array(w1165, w1161, w1152) -> (w1160:dbl[][])
    n788 = Reshape Array(w1199, w1161, w1152) -> (w1195:dbl[][])
    n789 = for {
      tunnel: w1158 -> [w1239] mode=indexing
      tunnel: [w1238] -> w1154 mode=indexing
      workers-P: _ -> [_]
      n790 = Add Array Elements(numeric array=w1239) -> (sum=w1238:dbl)
    }
    n791 = for {
      tunnel: w1157 -> [w1237] mode=indexing
      tunnel: [w1236] -> w1153 mode=indexing
      workers-P: _ -> [_]
      n792 = Add Array Elements(numeric array=w1237) -> (sum=w1236:dbl)
    }
    n793 = for {
      tunnel: w1192 -> [w1247] mode=indexing
      tunnel: [w1246] -> w1189 mode=indexing
      workers-P: _ -> [_]
      n794 = Add Array Elements(numeric array=w1247) -> (sum=w1246:dbl)
    }
    n795 = for {
      tunnel: w1191 -> [w1245] mode=indexing
      tunnel: [w1244] -> w1188 mode=indexing
      workers-P: _ -> [_]
      n796 = Add Array Elements(numeric array=w1245) -> (sum=w1244:dbl)
    }
    n797 = for {
      tunnel: w1159 -> [w1241] mode=indexing
      tunnel: [w1240] -> w1155 mode=indexing
      workers-P: _ -> [_]
      n798 = Add Array Elements(numeric array=w1241) -> (sum=w1240:dbl)
    }
    n799 = for {
      tunnel: w1193 -> [w1249] mode=indexing
      tunnel: [w1248] -> w1190 mode=indexing
      workers-P: _ -> [_]
      n800 = Add Array Elements(numeric array=w1249) -> (sum=w1248:dbl)
    }
    n801 = for {
      tunnel: w1160 -> [w1243] mode=indexing
      tunnel: [w1242] -> w1156 mode=indexing
      workers-P: _ -> [_]
      n802 = Add Array Elements(numeric array=w1243) -> (sum=w1242:dbl)
    }
    n803 = for {
      tunnel: w1195 -> [w1251] mode=indexing
      tunnel: [w1250] -> w1194 mode=indexing
      workers-P: _ -> [_]
      n804 = Add Array Elements(numeric array=w1251) -> (sum=w1250:dbl)
    }
    n805 = Divide(x=w1156, y=w1152) -> (x/y=w1121:dbl[])
    n806 = Divide(x=w1194, y=w1152) -> (x/y=w1123:dbl[])
    n807 = Divide(x=w1155, y=w1152) -> ()  [unwired: 1 out]
    n808 = Divide(x=w1154, y=w1152) -> (x/y=w1120:dbl[])
    n809 = Divide(x=w1190, y=w1152) -> ()  [unwired: 1 out]
    n810 = Divide(x=w1189, y=w1152) -> (x/y=w1122:dbl[])
    n811 = Divide(x=w1153, y=w1152) -> ()  [unwired: 1 out]
    n812 = Divide(x=w1188, y=w1152) -> ()  [unwired: 1 out]
    n813 = Build Array (concatenate)(w1120, w1141) -> (w1131:dbl[][])
    n814 = Build Array (concatenate)(w1120, w1148) -> (w1130:dbl[][])
    n815 = Build Array (concatenate)(w1121, w1138) -> (w1132:dbl[][])
    n816 = Build Array (concatenate)(w1121, w1146) -> (w1133:dbl[][])
    n817 = Build Array (concatenate)(w1122, w1214) -> (w1211:dbl[][])
    n818 = Build Array (concatenate)(w1122, w1215) -> (w1212:dbl[][])
    n819 = Build Array (concatenate)(w1123, w1216) -> (w1213:dbl[][])
    n820 = Build Array (concatenate)(w1123, w1220) -> (w1219:dbl[][])
    n821 = Reshape Array(w1131, w1137) -> (w1135:dbl[])
    n822 = Reshape Array(w1130, w1137) -> (w1134:dbl[])
    n823 = Reshape Array(w1132, w1137) -> (w1136:dbl[])
    n824 = Reshape Array(w1133, w1137) -> (w1145:dbl[])
    n825 = Reshape Array(w1211, w1137) -> (w1172:dbl[])
    n826 = Reshape Array(w1212, w1137) -> (w1173:dbl[])
    n827 = Reshape Array(w1213, w1137) -> (w1174:dbl[])
    n828 = Reshape Array(w1219, w1137) -> (w1175:dbl[])
    n829 = local read "Dis Sampling Rate"() -> (w1176:dbl)
    n830 = call-poly <vilib>:"Butterworth Filter.vi"("init/cont (init:F)"=TRUE, "order"=3, "filter type"="top filter", "low cutoff freq: fl"="fl Top", "high cutoff freq: fh"="fh Top", "sampling freq: fs"=w1176, "X"=w1175) -> ("Filtered X"=w1171:dbl[])  [unwired: 1 in, 1 out]
    n831 = call-poly <vilib>:"Butterworth Filter.vi"("init/cont (init:F)"=TRUE, "order"=3, "filter type"="bottom filter", "low cutoff freq: fl"="fl Bottom", "high cutoff freq: fh"="fh Bottom", "sampling freq: fs"=w1176, "X"=w1174) -> ("Filtered X"=w1204:dbl[])  [unwired: 1 in, 1 out]
    n832 = call-poly <vilib>:"Butterworth Filter.vi"("init/cont (init:F)"=TRUE, "order"=3, "filter type"="top filter", "low cutoff freq: fl"="fl Top", "high cutoff freq: fh"="fh Top", "sampling freq: fs"=w1176, "X"=w1145) -> ("Filtered X"=w1129:dbl[])  [unwired: 1 in, 1 out]
    n833 = call-poly <vilib>:"Butterworth Filter.vi"("init/cont (init:F)"=TRUE, "order"=3, "filter type"="bottom filter", "low cutoff freq: fl"="fl Bottom", "high cutoff freq: fh"="fh Bottom", "sampling freq: fs"=w1176, "X"=w1136) -> ("Filtered X"=w1128:dbl[])  [unwired: 1 in, 1 out]
    n834 = call-poly <vilib>:"Butterworth Filter.vi"("init/cont (init:F)"=TRUE, "order"=3, "filter type"="top filter", "low cutoff freq: fl"="fl Top", "high cutoff freq: fh"="fh Top", "sampling freq: fs"=w1176, "X"=w1173) -> ("Filtered X"=w1202:dbl[])  [unwired: 1 in, 1 out]
    n835 = call-poly <vilib>:"Butterworth Filter.vi"("init/cont (init:F)"=TRUE, "order"=3, "filter type"="top filter", "low cutoff freq: fl"="fl Top", "high cutoff freq: fh"="fh Top", "sampling freq: fs"=w1176, "X"=w1135) -> ("Filtered X"=w1127:dbl[])  [unwired: 1 in, 1 out]
    n836 = call-poly <vilib>:"Butterworth Filter.vi"("init/cont (init:F)"=TRUE, "order"=3, "filter type"="bottom filter", "low cutoff freq: fl"="fl Bottom", "high cutoff freq: fh"="fh Bottom", "sampling freq: fs"=w1176, "X"=w1172) -> ("Filtered X"=w1203:dbl[])  [unwired: 1 in, 1 out]
    n837 = call-poly <vilib>:"Butterworth Filter.vi"("init/cont (init:F)"=TRUE, "order"=3, "filter type"="bottom filter", "low cutoff freq: fl"="fl Bottom", "high cutoff freq: fh"="fh Bottom", "sampling freq: fs"=w1176, "X"=w1134) -> ("Filtered X"=w1126:dbl[])  [unwired: 1 in, 1 out]
    n838 = Build Array(w1171, w1204, w1202, w1203, w1129, w1128, w1127, w1126) -> (→"8 Ch Heart":dbl[][])
  }
  n839 = while {
    tunnel: w41 -> [w1258]
    tunnel: w32 -> [w1257]
    tunnel: w2 -> [w1253]
    stop <- FALSE stop-if-true
    n840 = Wait (ms)(milliseconds to wait=u32 100) -> ()  [unwired: 1 out]
    n841 = Get Queue Status(queue=w1258) -> (queue out=w1260:refnum<queue>, # elements in queue=w1261:i32)  [unwired: 2 in, 6 out]
    "# NCS Buffer" <- w1261
    n842 = Get Queue Status(queue=w1253) -> (queue out=w1254:refnum<queue>, # elements in queue=w1252:i32)  [unwired: 2 in, 6 out]
    n843 = local read "Save"() -> (w1255:bool)
    n844 = case shown="True" w1255 {
      tunnel: w1261 -> [_ w1330]
      tunnel: w1260 -> [_ w1331]
      tunnel: w1257 -> [_ w1329]
      tunnel: w1254 -> [_ w1270]
      tunnel: w1252 -> [_ w1265]
      frame False {
      }
      frame True {
        # "Once Saved: Stop saving"
        # "Getting channels from Buffer Queue"
        n845 = Multiply(x=w1330, y=w1329) -> (x*y=w1286:dbl)
        n846 = for {
          N: w1330 -> [_]
          tunnel: [w1523] -> w1302 mode=indexing
          tunnel: [w1519] -> w1301 mode=indexing
          tunnel: [w1518] -> w1299 mode=indexing
          tunnel: [w1517] -> w1297 mode=indexing
          shift-right: [w1515] -> _
          shift-left: w1331 -> [w1525]
          tunnel: [w1510] -> w1291 mode=indexing
          tunnel: [w1509] -> w1290 mode=indexing
          tunnel: [w1508] -> w1289 mode=indexing
          tunnel: [w1507] -> w1288 mode=indexing
          tunnel: [w1498] -> w1287 mode=indexing
          tunnel: [w1496] -> w1285 mode=indexing
          tunnel: [w1495] -> w1284 mode=indexing
          tunnel: [w1494] -> w1283 mode=indexing
          tunnel: [w1493] -> w1282 mode=indexing
          tunnel: [w1492] -> w1281 mode=indexing
          tunnel: [w1491] -> w1280 mode=indexing
          tunnel: [w1490] -> w1279 mode=indexing
          i -> [w1516]
          n847 = Dequeue Element(queue=w1525) -> (queue out=w1515:refnum<queue>, element=w1497:dbl[][])  [unwired: 2 in, 2 out]
          n848 = Index Array(array=w1497, index (row)=13) -> (element=w1492:dbl[])  [unwired: 1 in]
          n849 = Index Array(array=w1497, index (row)=14) -> (element=w1491:dbl[])  [unwired: 1 in]
          n850 = Index Array(array=w1497, index (row)=15) -> (element=w1490:dbl[])  [unwired: 1 in]
          n851 = Index Array(array=w1497, index (row)=9) -> (element=w1496:dbl[])  [unwired: 1 in]
          n852 = Index Array(array=w1497, index (row)=10) -> (element=w1495:dbl[])  [unwired: 1 in]
          n853 = Index Array(array=w1497, index (row)=11) -> (element=w1494:dbl[])  [unwired: 1 in]
          n854 = Index Array(array=w1497, index (row)=12) -> (element=w1493:dbl[])  [unwired: 1 in]
          n855 = Index Array(array=w1497, index (row)=5) -> (element=w1509:dbl[])  [unwired: 1 in]
          n856 = Index Array(array=w1497, index (row)=6) -> (element=w1508:dbl[])  [unwired: 1 in]
          n857 = Index Array(array=w1497, index (row)=7) -> (element=w1507:dbl[])  [unwired: 1 in]
          n858 = Index Array(array=w1497, index (row)=8) -> (element=w1498:dbl[])  [unwired: 1 in]
          n859 = Index Array(array=w1497, index (row)=4) -> (element=w1510:dbl[])  [unwired: 1 in]
          n860 = Index Array(array=w1497, index (row)=1) -> (element=w1519:dbl[])  [unwired: 1 in]
          n861 = Index Array(array=w1497, index (row)=2) -> (element=w1518:dbl[])  [unwired: 1 in]
          n862 = Index Array(array=w1497, index (row)=3) -> (element=w1517:dbl[])  [unwired: 1 in]
          n863 = Index Array(array=w1497, index (row)=0) -> (element=w1523:dbl[])  [unwired: 1 in]
          "NCS Save Loops" <- w1516
        }
        n864 = for {
          N: w1265 -> [_]
          tunnel: [w1340] -> w1267 mode=concatenating
          tunnel: [w1337] -> w1268 mode=concatenating
          tunnel: [w1336] -> w1269 mode=concatenating
          tunnel: w1270 -> [w1333]
          tunnel: [w1332] -> w1266 mode=concatenating
          n865 = Dequeue Element(queue=w1333) -> (element=w1334:dbl[][])  [unwired: 2 in, 3 out]
          n866 = Index Array(array=w1334, index (row)=0) -> (element=w1336:dbl[])  [unwired: 1 in]
          n867 = Index Array(array=w1334, index (row)=1) -> (element=w1337:dbl[])  [unwired: 1 in]
          n868 = Index Array(array=w1334, index (row)=2) -> (element=w1340:dbl[])  [unwired: 1 in]
          n869 = Index Array(array=w1334, index (row)=3) -> (element=w1332:dbl[])  [unwired: 1 in]
        }
        n870 = local read "Current Routine"() -> (w1328:string)
        n871 = local read "Case #"() -> (w1264:string)
        n872 = Concatenate Strings("Case", w1264, w1328) -> (w1262:string)
        n873 = flat-sequence {
          tunnel: w1304 -> [w1424]
          tunnel: w1305 -> [w1425]
          tunnel: w1306 -> [w1426]
          tunnel: w1307 -> [w1427]
          tunnel: w1308 -> [w1429]
          tunnel: w1309 -> [w1428]
          tunnel: w1310 -> [w1430]
          tunnel: w1311 -> [w1431]
          tunnel: w1312 -> [w1432]
          tunnel: w1313 -> [w1433]
          tunnel: w1314 -> [w1434]
          tunnel: w1315 -> [w1435]
          tunnel: w1316 -> [w1436]
          tunnel: w1317 -> [w1437]
          tunnel: "Abd (cm)" -> [w1459]
          tunnel: "Comments" -> [w1454]
          tunnel: "Weight (lbs)" -> [w1455]
          tunnel: "Thorax (cm)" -> [w1457]
          tunnel: "Height (cm)" -> [w1462]
          tunnel: "Age (yrs)" -> [w1464]
          tunnel: "Sex" -> [w1466]
          tunnel: "Case #" -> [w1467]
          tunnel: path "C:/Users/Edwin Kan Group/Documents/Zijing/dyspnea stuC:/Users/Edwin Kan Group/Documents/Zijing/dyspnea study/data/10_12" ("base path") -> [w1488]
          tunnel: w1262 -> [w1487]
          tunnel: w1303 -> [w1423]
          tunnel: w1296 -> [w1410]
          tunnel: w1298 -> [w1413]
          tunnel: w1300 -> [w1418]
          tunnel: w1295 -> [w1409]
          tunnel: w1294 -> [w1406]
          tunnel: w1293 -> [w1401]
          tunnel: w1292 -> [w1400]
          tunnel: w1278 -> [w1395]
          tunnel: w1277 -> [w1392]
          tunnel: w1276 -> [w1389]
          tunnel: w1275 -> [w1386]
          tunnel: w1274 -> [w1385]
          tunnel: w1273 -> [w1378]
          tunnel: w1272 -> [w1377]
          tunnel: w1271 -> [w1376]
          tunnel: w1269 -> [w1349]
          tunnel: w1268 -> [w1347]
          tunnel: w1267 -> [w1345]
          tunnel: w1266 -> [w1343]
          frame #0 {
            n874 = Build Path(base path=w1488, name or relative path=w1487) -> (appended path=w1470:path)
            n875 = TDMS Open(6:FALSE ("disable buffering (T)"), 10:T9."open or create" ("operation"), 11:w1470) -> (0:w1485:errorcluster, 3:w1486:refnum<k34>)  [unwired: 4 in]
            n876 = TDMS Set Properties(5:w1467, 7:"Case Number", 8:w1485, 11:w1486) -> (0:w1484:errorcluster, 3:w1483:refnum<k34>)  [unwired: 2 in, 2 out]
            n877 = TDMS Set Properties(5:w1466, 7:"Sex", 8:w1484, 11:w1483) -> (0:w1482:errorcluster, 3:w1481:refnum<k34>)  [unwired: 2 in, 2 out]
            n878 = TDMS Set Properties(5:w1464, 7:"Age (years)", 8:w1482, 11:w1481) -> (0:w1480:errorcluster, 3:w1479:refnum<k34>)  [unwired: 2 in, 2 out]
            n879 = TDMS Set Properties(5:w1462, 7:"Height (cm)", 8:w1480, 11:w1479) -> (0:w1477:errorcluster, 3:w1476:refnum<k34>)  [unwired: 2 in, 2 out]
            n880 = TDMS Set Properties(5:w1459, 7:"AbdCircumference (cm)", 8:w1477, 11:w1476) -> (0:w1475:errorcluster, 3:w1474:refnum<k34>)  [unwired: 2 in, 2 out]
            n881 = TDMS Set Properties(5:w1457, 7:"Thorax Circumference (cm)", 8:w1475, 11:w1474) -> (0:w1472:errorcluster, 3:w1473:refnum<k34>)  [unwired: 2 in, 2 out]
            n882 = TDMS Set Properties(5:w1455, 7:"Weight (lbs)", 8:w1472, 11:w1473) -> (0:w1456:errorcluster, 3:w1478:refnum<k34>)  [unwired: 2 in, 2 out]
            n883 = TDMS Set Properties(5:w1454, 7:"Comments", 8:w1456, 11:w1478) -> (0:w1438:errorcluster, 3:w1439:refnum<k34>)  [unwired: 2 in, 2 out]
            n884 = TDMS Set Properties(5:w1436, 7:w1437, 8:w1438, 11:w1439) -> (0:w1451:errorcluster, 3:w1450:refnum<k34>)  [unwired: 2 in, 2 out]
            n885 = TDMS Set Properties(5:w1434, 7:w1435, 8:w1451, 11:w1450) -> (0:w1449:errorcluster, 3:w1448:refnum<k34>)  [unwired: 2 in, 2 out]
            n886 = TDMS Set Properties(5:w1432, 7:w1433, 8:w1449, 11:w1448) -> (0:w1446:errorcluster, 3:w1445:refnum<k34>)  [unwired: 2 in, 2 out]
            n887 = TDMS Set Properties(5:w1430, 7:w1431, 8:w1446, 11:w1445) -> (0:w1444:errorcluster, 3:w1443:refnum<k34>)  [unwired: 2 in, 2 out]
            n888 = TDMS Set Properties(5:w1428, 7:w1429, 8:w1444, 11:w1443) -> (0:w1441:errorcluster, 3:w1442:refnum<k34>)  [unwired: 2 in, 2 out]
            n889 = TDMS Set Properties(5:w1426, 7:w1427, 8:w1441, 11:w1442) -> (0:w1440:errorcluster, 3:w1447:refnum<k34>)  [unwired: 2 in, 2 out]
            n890 = TDMS Set Properties(5:w1424, 7:w1425, 8:w1440, 11:w1447) -> (0:w1421:errorcluster, 3:w1422:refnum<k34>)  [unwired: 2 in, 2 out]
            n891 = TDMS Write(0:w1422, 7:"Tx1Rx1", 9:w1423, 11:w1421) -> (4:w1419:refnum<k34>, 15:w1420:errorcluster)  [unwired: 2 in, 2 out]
            n892 = TDMS Write(0:w1419, 7:"Tx2Rx1", 9:w1418, 11:w1420) -> (4:w1414:refnum<k34>, 15:w1415:errorcluster)  [unwired: 2 in, 2 out]
            n893 = TDMS Write(0:w1414, 7:"Tx3Rx1", 9:w1413, 11:w1415) -> (4:w1411:refnum<k34>, 15:w1412:errorcluster)  [unwired: 2 in, 2 out]
            n894 = TDMS Write(0:w1411, 7:"Tx4Rx1", 9:w1410, 11:w1412) -> (4:w1407:refnum<k34>, 15:w1408:errorcluster)  [unwired: 2 in, 2 out]
            n895 = TDMS Write(0:w1407, 7:"Tx1Rx2", 9:w1409, 11:w1408) -> (4:w1404:refnum<k34>, 15:w1405:errorcluster)  [unwired: 2 in, 2 out]
            n896 = TDMS Write(0:w1404, 7:"Tx2Rx2", 9:w1406, 11:w1405) -> (4:w1402:refnum<k34>, 15:w1403:errorcluster)  [unwired: 2 in, 2 out]
            n897 = TDMS Write(0:w1402, 7:"Tx3Rx2", 9:w1401, 11:w1403) -> (4:w1398:refnum<k34>, 15:w1399:errorcluster)  [unwired: 2 in, 2 out]
            n898 = TDMS Write(0:w1398, 7:"Tx4Rx2", 9:w1400, 11:w1399) -> (4:w1396:refnum<k34>, 15:w1397:errorcluster)  [unwired: 2 in, 2 out]
            n899 = TDMS Write(0:w1396, 7:"Tx1Rx3", 9:w1395, 11:w1397) -> (4:w1393:refnum<k34>, 15:w1394:errorcluster)  [unwired: 2 in, 2 out]
            n900 = TDMS Write(0:w1393, 7:"Tx2Rx3", 9:w1392, 11:w1394) -> (4:w1391:refnum<k34>, 15:w1388:errorcluster)  [unwired: 2 in, 2 out]
            n901 = TDMS Write(0:w1391, 7:"Tx3Rx3", 9:w1389, 11:w1388) -> (4:w1390:refnum<k34>, 15:w1387:errorcluster)  [unwired: 2 in, 2 out]
            n902 = TDMS Write(0:w1390, 7:"Tx4Rx3", 9:w1386, 11:w1387) -> (4:w1383:refnum<k34>, 15:w1384:errorcluster)  [unwired: 2 in, 2 out]
            n903 = TDMS Write(0:w1383, 7:"Tx1Rx4", 9:w1385, 11:w1384) -> (4:w1382:refnum<k34>, 15:w1381:errorcluster)  [unwired: 2 in, 2 out]
            n904 = TDMS Write(0:w1382, 7:"Tx2Rx4", 9:w1378, 11:w1381) -> (4:w1379:refnum<k34>, 15:w1380:errorcluster)  [unwired: 2 in, 2 out]
            n905 = TDMS Write(0:w1379, 7:"Tx3Rx4", 9:w1377, 11:w1380) -> (4:w1374:refnum<k34>, 15:w1375:errorcluster)  [unwired: 2 in, 2 out]
            n906 = TDMS Write(0:w1374, 7:"Tx4Rx4", 9:w1376, 11:w1375) -> (4:w1359:refnum<k34>, 15:w1354:errorcluster)  [unwired: 2 in, 2 out]
            n907 = TDMS Write(0:w1359, 7:"BIOPAC_CH1", 9:w1349, 11:w1354) -> (4:w1358:refnum<k34>, 15:w1353:errorcluster)  [unwired: 2 in, 2 out]
            n908 = TDMS Write(0:w1358, 7:"BIOPAC_CH2", 9:w1347, 11:w1353) -> (4:w1357:refnum<k34>, 15:w1352:errorcluster)  [unwired: 2 in, 2 out]
            n909 = TDMS Write(0:w1357, 7:"BIOPAC_CH3", 9:w1345, 11:w1352) -> (4:w1356:refnum<k34>, 15:w1351:errorcluster)  [unwired: 2 in, 2 out]
            n910 = TDMS Write(0:w1356, 7:"BIOPAC_CH4", 9:w1343, 11:w1351) -> (4:w1355:refnum<k34>, 15:w1350:errorcluster)  [unwired: 2 in, 2 out]
            n911 = TDMS Close(8:w1350, 11:w1355) -> ()  [unwired: 2 out]
          }
          frame #1 {
            n912 = local write "Save"(FALSE) -> ()
          }
        }
        n913 = local read "Start Time"() -> (w1320:T2)
        n914 = property on="fractional second" class="DigNum (strict)"() -> ("Label.Text"=w1317:string)  [unwired: 2 in, 2 out]
        n915 = property on="second" class="DigNum (strict)"() -> ("Label.Text"=w1315:string)  [unwired: 2 in, 2 out]
        n916 = Unbundle By Name(w1320) -> ("fractional second"=w1316:dbl, "second"=w1314:i32, "minute"=w1312:i32, "hour"=w1310:i32, "day of month"=w1309:i32, "month"=w1306:i32, "year"=w1304:i32)
        n917 = property on="minute" class="DigNum (strict)"() -> ("Label.Text"=w1313:string)  [unwired: 2 in, 2 out]
        n918 = property on="hour" class="DigNum (strict)"() -> ("Label.Text"=w1311:string)  [unwired: 2 in, 2 out]
        n919 = property on="month" class="DigNum (strict)"() -> ("Label.Text"=w1307:string)  [unwired: 2 in, 2 out]
        n920 = property on="day of month" class="DigNum (strict)"() -> ("Label.Text"=w1308:string)  [unwired: 2 in, 2 out]
        n921 = property on="year" class="DigNum (strict)"() -> ("Label.Text"=w1305:string)  [unwired: 2 in, 2 out]
        n922 = Reshape Array(w1302, w1286) -> (w1303:dbl[])
        n923 = Reshape Array(w1301, w1286) -> (w1300:dbl[])
        n924 = Reshape Array(w1299, w1286) -> (w1298:dbl[])
        n925 = Reshape Array(w1297, w1286) -> (w1296:dbl[])
        n926 = Reshape Array(w1291, w1286) -> (w1295:dbl[])
        n927 = Reshape Array(w1290, w1286) -> (w1294:dbl[])
        n928 = Reshape Array(w1289, w1286) -> (w1293:dbl[])
        n929 = Reshape Array(w1288, w1286) -> (w1292:dbl[])
        n930 = Reshape Array(w1287, w1286) -> (w1278:dbl[])
        n931 = Reshape Array(w1285, w1286) -> (w1277:dbl[])
        n932 = Reshape Array(w1284, w1286) -> (w1276:dbl[])
        n933 = Reshape Array(w1283, w1286) -> (w1275:dbl[])
        n934 = Reshape Array(w1282, w1286) -> (w1274:dbl[])
        n935 = Reshape Array(w1281, w1286) -> (w1273:dbl[])
        n936 = Reshape Array(w1280, w1286) -> (w1272:dbl[])
        n937 = Reshape Array(w1279, w1286) -> (w1271:dbl[])
      }
    }
  }
  n938 = while {
    stop <- FALSE stop-if-true
    # "Viewing NCS"
    n939 = local read "8 Ch Heart"() -> (w1533:dbl[][])
    n940 = Index Array(array=w1533, index (row)=6 ("index")) -> (element=→"Tx4Rx4":dbl[])  [unwired: 1 in]
    n941 = Index Array(array=w1533, index (row)=7 ("index")) -> (element=→"Tx3Rx4":dbl[])  [unwired: 1 in]
    n942 = Index Array(array=w1533, index (row)=3 ("index")) -> (element=→"Tx1Rx2":dbl[])  [unwired: 1 in]
    n943 = Index Array(array=w1533, index (row)=2 ("index")) -> (element=→"Tx2Rx2":dbl[])  [unwired: 1 in]
    n944 = Index Array(array=w1533, index (row)=0 ("index")) -> (element=→"Tx1Rx1":dbl[])  [unwired: 1 in]
    n945 = Index Array(array=w1533, index (row)=5 ("index")) -> (element=→"Tx4Rx3":dbl[])  [unwired: 1 in]
    n946 = Index Array(array=w1533, index (row)=4 ("index")) -> (element=→"Tx3Rx3":dbl[])  [unwired: 1 in]
    n947 = Index Array(array=w1533, index (row)=1 ("index")) -> (element=→"Tx2Rx1":dbl[])  [unwired: 1 in]
    n948 = Wait (ms)(milliseconds to wait=u32 30) -> ()  [unwired: 1 out]
  }
  "error out 1" <- w169
  "error out 2" <- w103
  "DownSamplingRatio" <- "DownSamplingRatio1"
  "ACQ ms" <- 100.0
  "Connecting" <- w1
  "Stopping" <- w1
  "Disconnecting" <- w1
  "Boolean" <- TRUE
  "Disconnected" <- w1
  "Connected" <- w1
  "Receive Success" <- w1
  "Receiving" <- w1
  "Acq Started" <- w1
